vi "Alicat Full Driver Example.vi"() -> ()   [LabVIEW 2020]
doc: "Example program displaying the potential usage of nearly all of the VI's included in the Alicat LabVIEW Driver Library.\n\nThis VI only connects to a single Alicat at a time, and some features may be locked out due to circuit board revision or firmware revision (newer units have additional features available to them).\n\nIf you have any questions regarding the VI's used in this example, please see the Alicat LabVIEW Driver Library Manual (available on the Alicat website and included in the driver library. If you have remaining questions, please contact Alicat at (520) 290-6060 or info@alicat.com."
panel:
  in  "Tare AP Sensor":bool
  in  "Wait message":cluster{"Boolean":bool}
  in  "Read/Write Options":T1 {"Controller Select" items=["No controller"=0, "Volumetric Flow"=36, "Mass Flow"=37, "Absolute Pressure"=34, "Gauge Pressure"=38, "Differential Pressure"=39]}
  out "Batch Units":string="SL"
  in  "Serial Only":T2={"Valve Drive"=FALSE, "Totalizer"=TRUE, "Totalizer Timer"=FALSE, "Totalizer Peak Flow"=FALSE, "Show Abs., Gauge\nand Baro. pressures"=FALSE}
  in  "Data Logging Options":T3={"Absolute Press."=TRUE, "Gauge/Diff. Press."=TRUE, "Barometric Press."=TRUE, "Temperature"=TRUE, "Volumetric"=TRUE, "Mass Flow"=TRUE, "Setpoint"=TRUE, "Valve Drive"=FALSE, "Totalizer"=TRUE, "Tot. Timer [s]"=FALSE, "Tot. Avg. Flow"=FALSE, "Tot. Peak Flow"=FALSE, "Gas Selected"=TRUE, "Log Data"=FALSE}
  out "Measurement Data":T4
  in  "Chart: Manual Scale Adjust":bool
  in  "Chart: AutoScale":bool=TRUE
  out "Chart":T5(graph)
  out "Register value":string
  in  "Reg. to read":u16
  in  "Read Register":bool
  in  "COMPOSER gas mix input":T6={"Mix % 1"=0.0, "Include # 1"=FALSE, "Mix % 2"=0.0, "Include # 2"=FALSE, "Mix % 3"=0.0, "Include # 3"=FALSE, "Mix % 4"=0.0, "Include # 4"=FALSE, "Mix % 5"=0.0, "Include # 5"=FALSE, "COMPOSER gas 1"=0, "COMPOSER gas 2"=0, "COMPOSER gas 3"=0, "COMPOSER gas 4"=0, "COMPOSER gas 5"=0, "Create COMPOSER Mix"=FALSE, "Mix #"=236, "Mix name"="MyMix1", "Completion\ntext"="", "Create COMPOSER Mix 2"=FALSE} {"Mix #" min=236 max=255 step=1; "Mix % 1" min=0.0 max=100.0 step=0.01; "Mix % 2" min=0.0 max=100.0 step=0.01; "Mix % 3" min=0.0 max=100.0 step=0.01; "Mix % 4" min=0.0 max=100.0 step=0.01; "Mix % 5" min=0.0 max=100.0 step=0.01}
  in  "Chart: Setpoint":bool=TRUE
  in  "PID Settings":T7 {"P Gain" min=0 max=65535 step=1; "D Gain" min=0 max=65535 step=1; "I Gain" min=0 max=65535 step=1}
  in  "Log Register Values":bool
  out "Meas. per\nsecond [Hz]":dbl caption="Elapsed Time (s)"
  out "Time between\nreadings [ms]":dbl caption="Elapsed Time (s)"
  in  "Chart: Graphing":bool=TRUE
  out "Read-Only Options":T8={"Analog SP"=enum."4-20mA", "Control Invert"=enum."Pressure", "Main PWM"=enum."Volumetric Flow 0-2.5-5V bidir", "Aux PWM"=enum."Fixed 0.00V"}
  in  "Tare Options":T9={"Display"=enum."None", "External"=enum."None", "Auto-Tare Delay [s]"=nan} {"Auto-Tare Delay [s]" min=0.0 max=25.5 step=0.1 format="%.1g"}
  in  "Tare Pressure":bool
  in  "Tare Flow":bool
  in  "Reset Total":bool
  in  "Chart: Mass Flow":bool=TRUE
  in  "Chart: Volumetric":bool=TRUE
  in  "Chart: Temperature":bool=TRUE
  in  "Chart: Pressure":bool=TRUE
  in  "Time between \nreadings [ms]":u32
  out "Totalizer":T10(ring)
  out "Setpoint Units":string="SLPM"
  in  "Serial and Display":T11={"Pressure"=TRUE, "Temperature"=TRUE, "Volumetric"=TRUE, "Mass Flow"=TRUE, "Tot. Avg Flow"=FALSE, "Gas Selected"=TRUE}
  out "(Full Scale)":dbl=nan
  in  "Setpoint":dbl
  in  "Batch Setpoint":dbl format="%.3f"
  in  "Gas Select":u16(ring)
  out "Manufacturer Info":string
  in  "COM Port Settings":T12={"Unit ID"="A", "Baud Rate"=enum."19200", "VISA Sesssion In"="COM1"}
  # "Setpoint and Batching Controls"
  # "Manual Tare"
  # "Data Frame Enables"
  # "Controller Options\nand Analog Signal\nInformation"
  # "(Resetting the Totalizer will reset the batch)"
  # "Graphing Options:"
  # "VI Timing Options"
  # "Register Values"
  # "Populating VI with device information, please wait."
  # "Altering log options will start a new data log"
  # "(The data will be logged to the folder containing the VI)"
  # "Totalizer Timer"
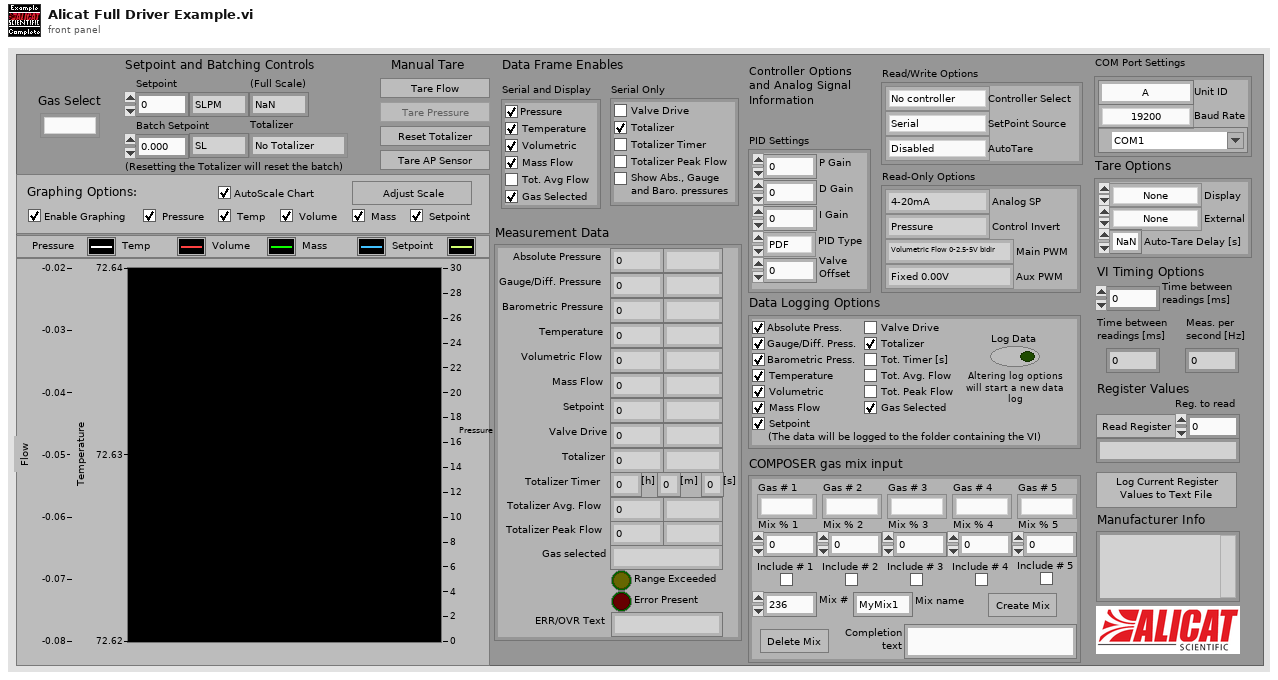
[diagram p1: front panel]
types:
  T1 = cluster{"Controller Select":u16, "SetPoint Source":enum8{"Serial", "Local", "Analog", "Unknown"}, "AutoTare":enum16{"Disabled", "Enabled"}}
  T2 = cluster{"Valve Drive":bool, "Totalizer":bool, "Totalizer Timer":bool, "Totalizer Peak Flow":bool, "Show Abs., Gauge\nand Baro. pressures":bool}
  T3 = cluster{"Absolute Press.":bool, "Gauge/Diff. Press.":bool, "Barometric Press.":bool, "Temperature":bool, "Volumetric":bool, "Mass Flow":bool, "Setpoint":bool, "Valve Drive":bool, "Totalizer":bool, "Tot. Timer [s]":bool, "Tot. Avg. Flow":bool, "Tot. Peak Flow":bool, "Gas Selected":bool, "Log Data":bool}
  T4 = cluster{"Absolute Pressure":dbl, "Gauge/Diff. Pressure":dbl, "Barometric Pressure":dbl, "Temperature":dbl, "Volumetric Flow":dbl, "Mass Flow":dbl, "Setpoint":dbl, "Valve Drive":dbl, "Totalizer":dbl, "[h]":dbl, "[m]":dbl, "[s]":dbl, "Totalizer Avg. Flow":dbl, "Totalizer Peak Flow":dbl, "Gas selected":string, "Range Exceeded":bool, "Error Present":bool, "ERR/OVR Text":string, "Abs. Pressure":string, "Temperature 2":string, "Volume":string, "Mass":string, "Totalizer 2":string, "Valve Drive 2":string, "Gauge/Diff. Press.":string, "Barometric Press.":string, "Setpoint 2":string, "Tot. Avg. Flow":string, "Tot. Peak Flow":string}
  T5 = cluster{"Pressure":dbl, "Temperature":dbl, "Volumetric":dbl, "Mass":dbl, "SetPoint":dbl}
  T6 = cluster{"Mix % 1":dbl, "Include # 1":bool, "Mix % 2":dbl, "Include # 2":bool, "Mix % 3":dbl, "Include # 3":bool, "Mix % 4":dbl, "Include # 4":bool, "Mix % 5":dbl, "Include # 5":bool, "COMPOSER gas 1":u16, "COMPOSER gas 2":u16, "COMPOSER gas 3":u16, "COMPOSER gas 4":u16, "COMPOSER gas 5":u16, "Create COMPOSER Mix":bool, "Mix #":u16, "Mix name":string, "Completion\ntext":string, "Create COMPOSER Mix 2":bool}
  T7 = cluster{"P Gain":i32, "D Gain":i32, "I Gain":i32, "PID Type":enum8{"PDF", "PD2I"}, "Valve \nOffset":i32}
  T8 = cluster{"Analog SP":enum16{"0-5V", "4-20mA"}, "Control Invert":enum16{"Pressure", "Vacuum/BP"}, "Main PWM":enum8{"Fixed 0.00V", "Pressure 0-5V", "Temperature 0-5V", "Volumetric Flow 0-5V", "Mass Flow 0-5V", "Pressure 0-2.5-5V bidir", "Temperature 0-2.5-5V bidir", "Volumetric Flow 0-2.5-5V bidir", "Mass Flow 0-2.5-5V bidir", "Pressure 1-5V", "Temperature 1-5V", "Volumetric Flow 1-5V", "Mass Flow 1-5V", "Reserved(A)", "Reserved(B)", "Fixed 5.12V"}, "Aux PWM":enum8{"Fixed 0.00V", "Pressure 0-5V", "Temperature 0-5V", "Volumetric Flow 0-5V", "Mass Flow 0-5V", "Pressure 0-2.5-5V bidir", "Temperature 0-2.5-5V bidir", "Volumetric Flow 0-2.5-5V bidir", "Mass Flow 0-2.5-5V bidir", "Pressure 1-5V", "Temperature 1-5V", "Volumetric Flow 1-5V", "Mass Flow 1-5V", "Reserved(A)", "Reserved(B)", "Fixed 5.12V"}}
  T9 = cluster{"Display":enum16{"None", "Pressure", "Volumetric"}, "External":enum16{"None", "Pressure", "Volumetric", "Totalizer"}, "Auto-Tare Delay [s]":dbl}
  T10 = enum8{"No Totalizer", "Mass Flow", "Volumetric Flow"}
  T11 = cluster{"Pressure":bool, "Temperature":bool, "Volumetric":bool, "Mass Flow":bool, "Tot. Avg Flow":bool, "Gas Selected":bool}
  T12 = cluster{"Unit ID":string, "Baud Rate":enum8{"2400", "9600", "19200", "38400", "57600", "115200", "Unknown"}, "VISA Sesssion In":refnum<visa-resource-name>}
  T13 = cluster{"Absolute Pressure":bool, "Gauge/Diff. Pressure":bool, "Barometric Pressure":bool, "Temperature":bool, "Volumetric":bool, "Mass":bool, "Setpoint":bool, "Valve Drive":bool, "Totalizer":bool, "Totalizer Timer":bool, "Totalizer Average Flow":bool, "Totalizer Peak Flow":bool, "Gas Selected":bool, "Tot. Timer Format":u16}
  T14 = cluster{"Controller Full Scale":dbl, "Controller Select":u16, "Control Range":enum16{"Normal", "Inverted", "Bidirectional", "Unknown"}}
  T15 = cluster{"Absolute Pressure":dbl, "Gauge/Diff. Pressure":dbl, "Barometric Pressure":dbl, "Temperature":dbl, "Volumetric Flow":dbl, "Mass Flow":dbl, "Setpoint":dbl, "Valve Drive":dbl, "Totalizer":dbl, "[h]":dbl, "[m]":dbl, "[s]":dbl, "Totalizer Average Flow":dbl, "Totalizer Peak Flow":dbl, "Gas selected":string, "Range Exceeded":bool, "Error Present":bool, "ERR/OVR Text":string, "Abs. Pressure":string, "Temperature 2":string, "Volume":string, "Mass":string, "Totalizer 2":string, "Valve Drive 2":string, "Gauge/Diff. Press.":string, "Barometric Press.":string, "Setpoint 2":string, "Tot. Avg. Flow":string, "Tot. Peak Flow":string}
  T16 = cluster{"Abs. Pressure":string, "Gauge/Diff. Press.":string, "Barometric Press.":string, "Temperature":string, "Volume":string, "Mass":string, "Setpoint":string, "Valve Drive":string, "Totalizer":string, "Tot. Timer":string, "Tot. Avg. Flow":string, "Tot. Peak Flow":string}
  T17 = cluster{"Pressure":bool, "Temperature":bool, "Volumetric":bool, "Mass Flow":bool, "Setpoint":bool, "Chart: AutoScale":bool}
  T18 = cluster{"Enabled":enum8{"Enabled", "Disabled", "Disabled and Grayed Out"}, "Disabled and Grayed Out":enum8{"Enabled", "Disabled", "Disabled and Grayed Out"}}
  T19 = cluster{"Absolute Pressure":dbl, "Gauge/Diff. Pressure":dbl, "Barometric Pressure":dbl, "Temperature":dbl, "Volumetric":dbl, "Mass Flow":dbl, "Setpoint":dbl, "Valve Drive":dbl, "Totalizer":dbl, "[hr]":dbl, "[min]":dbl, "[sec]":dbl, "Totalizer Average Flow":dbl, "Totalizer Peak Flow":dbl, "Gas selected":string}
  T20 = cluster{"Pressure(s)":bool, "Temperature":bool, "Volumetric":bool, "Mass":bool, "Totalizer Average Flow":bool, "Gas Selected":bool}
  T21 = enum16{"open", "replace", "create", "open or create", "replace or create", "replace or create with confirmation"}
  T22 = cluster{"P Gain":i32, "D Gain":i32, "I Gain":i32}
  T23 = cluster{"PID Type":enum8{"PDF", "PD2I"}, "Valve Offset":i32}
  T24 = cluster{"Gas # 1":u16, "Mix % 1":dbl, "Include # 1":bool, "Gas # 2":u16, "Mix % 2":dbl, "Include # 2":bool, "Gas # 3":u16, "Mix % 3":dbl, "Include # 3":bool, "Gas # 4":u16, "Mix % 4":dbl, "Include # 4":bool, "Gas # 5":u16, "Mix % 5":dbl, "Include # 5":bool}
  T25 = cluster{"Pressure":bool, "Temperature":bool, "Volumetric":bool, "Mass":bool, "Totalizer Average Flow":bool, "Gas Selected":bool}
  T26 = enum8{"Enabled", "Disabled", "Disabled and Grayed Out"}
  T27 = typedef "Data Frame.ctl" = cluster{"Absolute Pressure":bool, "Gauge/Diff. Pressure":bool, "Barometric Pressure":bool, "Temperature":bool, "Volumetric":bool, "Mass":bool, "Setpoint":bool, "Valve Drive":bool, "Totalizer":bool, "Totalizer Timer":bool, "Totalizer Average Flow":bool, "Totalizer Peak Flow":bool, "Gas Selected":bool, "Tot. Timer Format":u16}
  T28 = enum16{"None", "Pressure", "Volumetric", "Totalizer"}
  T29 = cluster{"Valve Amount":enum8{"Single Valve", "Dual Valve"}, "PID Type":enum8{"PDF", "PD2I"}, "Valve Offset":i32, "P Gain":i32, "D Gain":i32, "I Gain":i32}
  T30 = cluster{"Absolute Pressure":dbl, "Gauge/Diff. Pressure":dbl, "Volumetric Flow":dbl, "Mass Flow":dbl}
  T31 = typedef "Data Cluster.ctl" = cluster{"Absolute Pressure":dbl, "Gauge/Diff. Pressure":dbl, "Barometric Pressure":dbl, "Temperature":dbl, "Volumetric Flow":dbl, "Mass Flow":dbl, "Setpoint":dbl, "Valve Drive":dbl, "Totalizer":dbl, "[hr]":dbl, "[min]":dbl, "[sec]":dbl, "Totalizer Average Flow":dbl, "Totalizer Peak Flow":dbl, "Gas selected":string}
  T32 = enum8{"2400", "9600", "19200", "38400", "57600", "115200", "Unknown"}
  T33 = cluster{"Absolute Pressure":dbl, "Gauge/Diff. Pressure":dbl, "Barometric Pressure":dbl, "Temperature":dbl, "Volumetric Flow":dbl, "Mass Flow":dbl, "Setpoint":dbl, "Valve Drive":dbl, "Totalizer":dbl, "[hr]":dbl, "[min]":dbl, "[sec]":dbl, "Totalizer Average Flow":dbl, "Totalizer Peak Flow":dbl, "Gas selected":string}
  T34 = cluster{"Pressure":bool, "Temperature":bool, "Volumetric":bool, bool, bool, "Gas Selected":bool}
  T35 = enum16{"Left Button", "Center Button", "Right Button", "Window Close"}
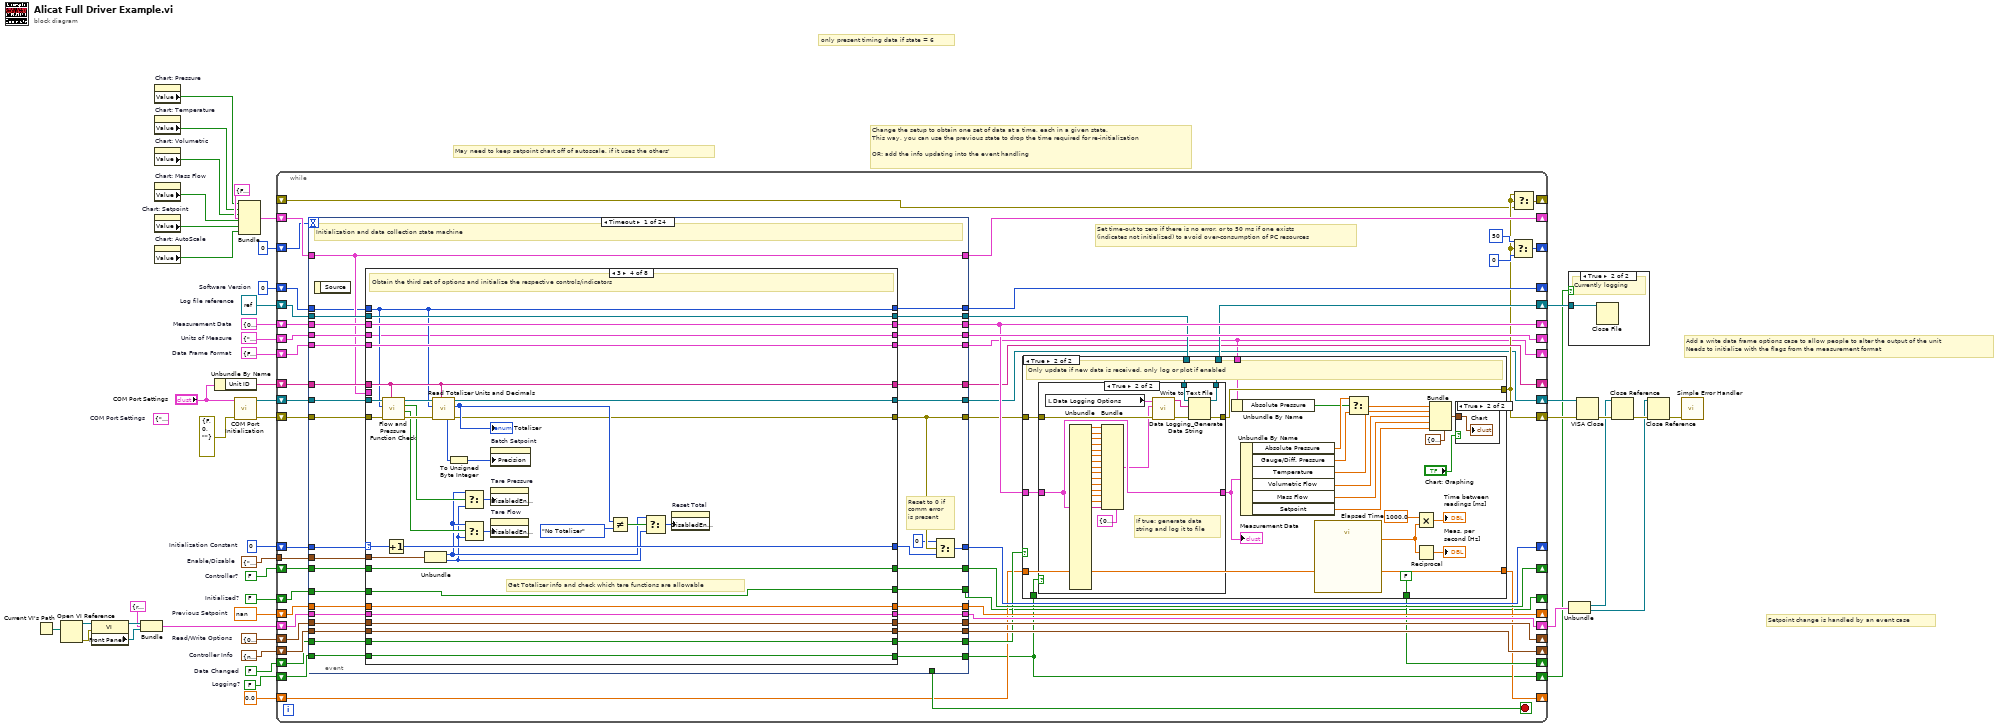
[diagram p0: block diagram]
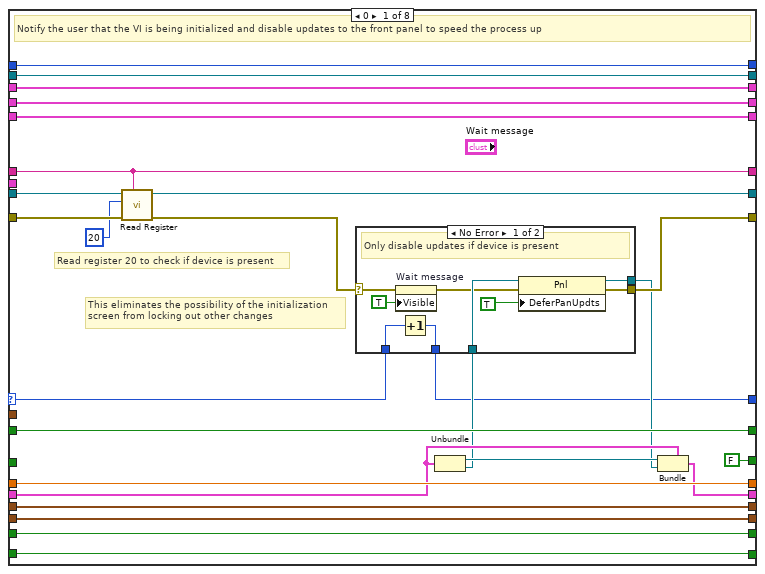
[diagram p6: hidden frame]
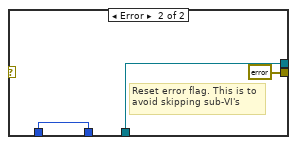
[diagram p7: hidden frame]
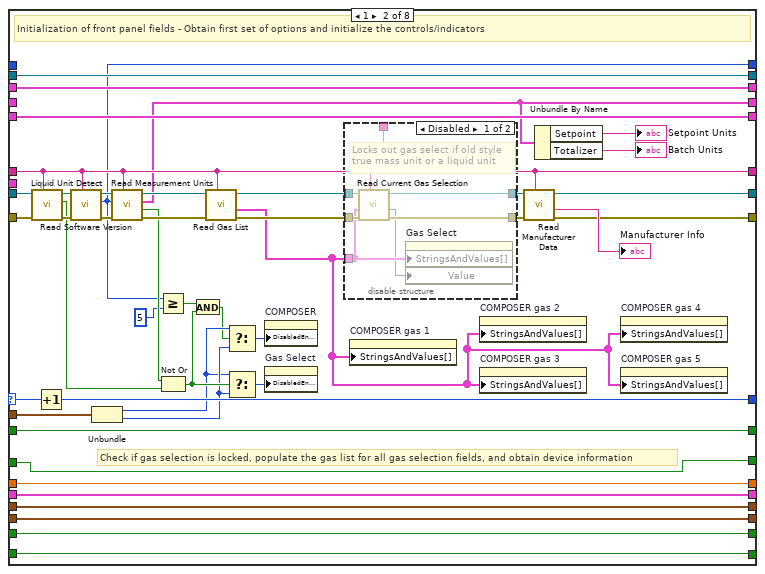
[diagram p8: hidden frame]
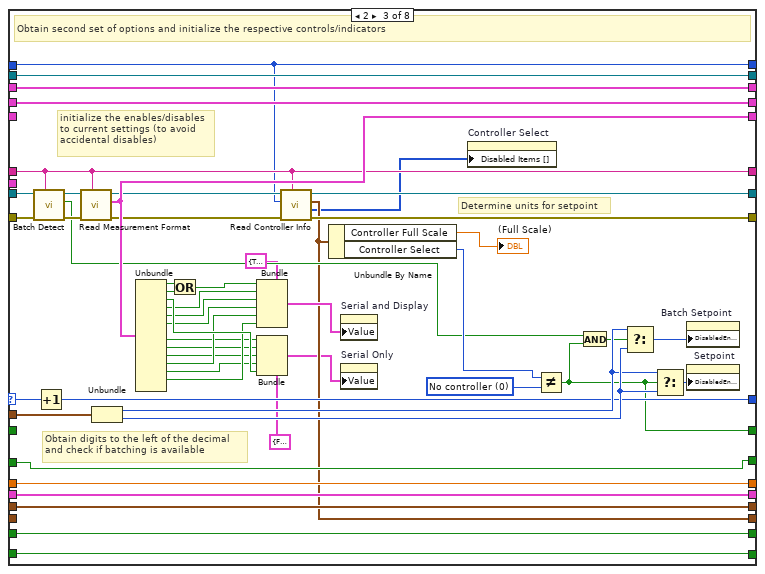
[diagram p10: hidden frame]
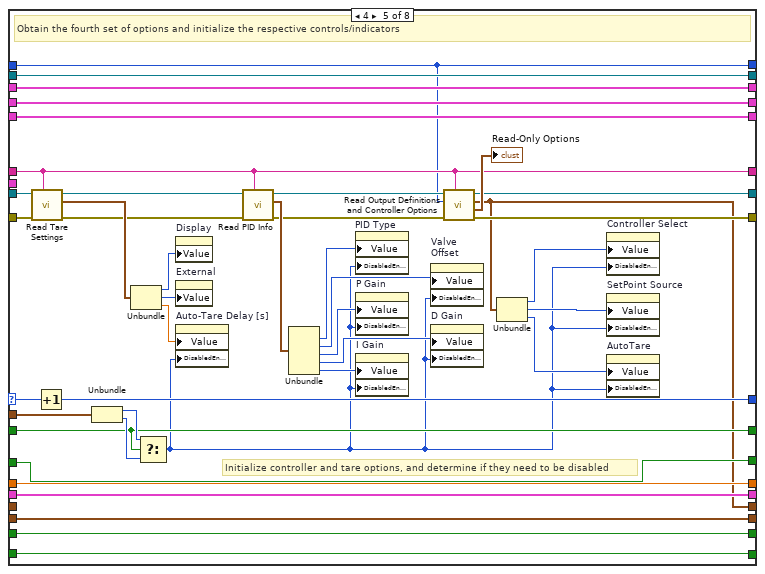
[diagram p11: hidden frame]
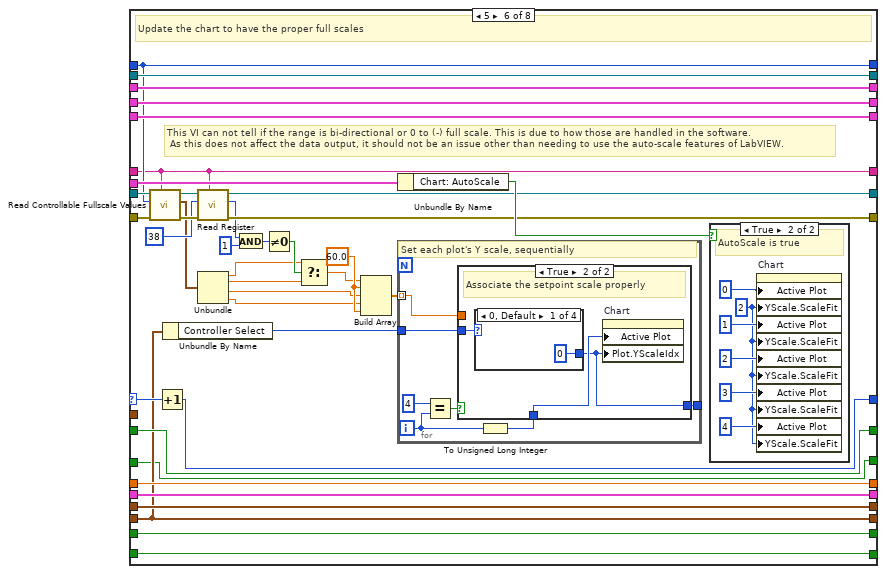
[diagram p12: hidden frame]
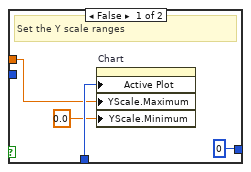
[diagram p14: hidden frame]
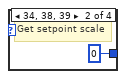
[diagram p15: hidden frame]
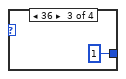
[diagram p16: hidden frame]
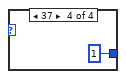
[diagram p17: hidden frame]
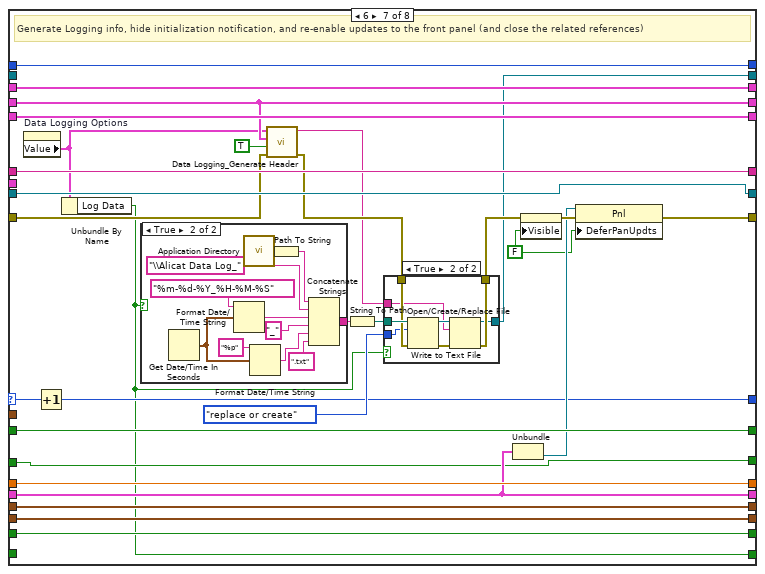
[diagram p18: hidden frame]
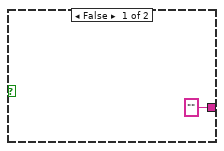
[diagram p19: hidden frame]
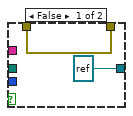
[diagram p20: hidden frame]
diagram:
  w1 = T13 {"Absolute Pressure"=FALSE, "Gauge/Diff. Pressure"=FALSE, "Barometric Pressure"=FALSE, "Temperature"=FALSE, "Volumetric"=FALSE, "Mass"=FALSE, "Setpoint"=FALSE, "Valve Drive"=FALSE, "Totalizer"=FALSE, "Totalizer Timer"=FALSE, "Totalizer Average Flow"=FALSE, "Totalizer Peak Flow"=FALSE, "Gas Selected"=FALSE, "Tot. Timer Format"=0}  # Data Frame Format
  w2 = T1 {"Controller Select"=0, "SetPoint Source"=enum."Serial", "AutoTare"=enum."Disabled"}  # Read/Write Options
  w3 = T14 {"Controller Full Scale"=nan, "Controller Select"=0, "Control Range"=enum."Normal"}  # Controller Info
  (unwired) T12 {"Unit ID"="A", "Baud Rate"=enum."19200", "VISA Sesssion In"="COM1"}  # COM Port Settings
  w4 = T15 {"Absolute Pressure"=0.0, "Gauge/Diff. Pressure"=0.0, "Barometric Pressure"=0.0, "Temperature"=0.0, "Volumetric Flow"=0.0, "Mass Flow"=0.0, "Setpoint"=0.0, "Valve Drive"=0.0, "Totalizer"=0.0, "[h]"=0.0, "[m]"=0.0, "[s]"=0.0, "Totalizer Average Flow"=0.0, "Totalizer Peak Flow"=0.0, "Gas selected"="", "Range Exceeded"=FALSE, "Error Present"=FALSE, "ERR/OVR Text"="", "Abs. Pressure"="", "Temperature 2"="", "Volume"="", "Mass"="", "Totalizer 2"="", "Valve Drive 2"="", "Gauge/Diff. Press."="", "Barometric Press."="", "Setpoint 2"="", "Tot. Avg. Flow"="", "Tot. Peak Flow"=""}  # Measurement Data
  w5 = T16 {"Abs. Pressure"="", "Gauge/Diff. Press."="", "Barometric Press."="", "Temperature"="", "Volume"="", "Mass"="", "Setpoint"="", "Valve Drive"="", "Totalizer"="", "Tot. Timer"="", "Tot. Avg. Flow"="", "Tot. Peak Flow"=""}  # Units of Measure
  w6 = u8 0  # Software Version
  w8 = FALSE  # Logging?
  w9 = FALSE  # Initialized?
  w25 = FALSE  # Data Changed
  w27 = refnum<file> refnum  # Log file reference
  w37 = nan  # Previous Setpoint
  w38 = FALSE  # Controller?
  w39 = T18 {"Enabled"=enum."Enabled", "Disabled and Grayed Out"=enum."Disabled and Grayed Out"}  # Enable/Disable
  w40 = 0  # Initialization Constant
  # "May need to keep setpoint chart off of autoscale, if it uses the others'"
  # "only present timing data if state = 6"
  # "Change the setup to obtain one set of data at a time, each in a given state.\nThis way, you can use the previous state to drop the time required for re-initialization\n\nOR: add the info updating into the event handling"
  # "Setpoint change is handled by an event case"
  # "Add a write data frame options case to allow people to alter the output of the unit\nNeeds to initialize with the flags from the measurement format"
  n1 = Current VI's Path() -> (path=w34:path)
  n2 = Open VI Reference(vi path=w34) -> (vi reference=w32:refnum<vi>, error out=w33:errorcluster)  [unwired: 2 in, 3 out]
  n3 = property class="VI"(reference=w32, error in=w33) -> (reference out=w30:refnum<vi>, "Front Panel"=w31:refnum<vi>)  [unwired: 1 out]
  n4 = Bundle(cluster=cluster{refnum<vi>, "Panel":refnum<vi>} {refnum, "Panel"=refnum}, w30, "Panel"=w31) -> (w29:cluster{refnum<vi>, "Panel":refnum<vi>})
  n5 = property on="Chart: Pressure" class="Bool (strict)"() -> ("Value"=w19:bool)  [unwired: 2 in, 2 out]
  n6 = property on="Chart: Temperature" class="Bool (strict)"() -> ("Value"=w20:bool)  [unwired: 2 in, 2 out]
  n7 = property on="Chart: Volumetric" class="Bool (strict)"() -> ("Value"=w21:bool)  [unwired: 2 in, 2 out]
  n8 = property on="Chart: Mass Flow" class="Bool (strict)"() -> ("Value"=w22:bool)  [unwired: 2 in, 2 out]
  n9 = property on="Chart: Setpoint" class="Bool (strict)"() -> ("Value"=w23:bool)  [unwired: 2 in, 2 out]
  n10 = property on="Chart: AutoScale" class="Bool (strict)"() -> ("Value"=w17:bool)  [unwired: 2 in, 2 out]
  n11 = Unbundle By Name("COM Port Settings") -> ("Unit ID"=w41:string)
  n12 = call "COM Port Initialization.vi"("error in (no error)"=errorcluster {"status"=FALSE, "code"=0, "source"=""}, "Communication Settings"="COM Port Settings") -> ("error out"=w44:errorcluster, "VISA Session Out"=w46:refnum<visa-resource-name>)  [unwired: 8 in]
  n13 = Bundle(cluster=T17 {"Pressure"=FALSE, "Temperature"=FALSE, "Volumetric"=FALSE, "Mass Flow"=FALSE, "Setpoint"=FALSE, "Chart: AutoScale"=TRUE} ("Graphing enables"), "Pressure"=w19, "Temperature"=w20, "Volumetric"=w21, "Mass Flow"=w22, "Setpoint"=w23, "Chart: AutoScale"=w17) -> (w35:T17)
  n14 = while {
    shift-right: [w91] -> _
    shift-left: w40 -> [w92]
    shift-right: [w73] -> _
    shift-left: w4 -> [w90]
    shift-right: [w88] -> _
    shift-left: w5 -> [w89]
    tunnel: w39 -> [w87]
    shift-right: [w47] -> _
    shift-left: w1 -> [w86]
    shift-right: [w48] -> w45
    shift-left: w46 -> [w95]
    shift-right: [w51] -> w43
    shift-left: w44 -> [w94]
    shift-right: [w52] -> _
    shift-left: w41 -> [w93]
    shift-right: [w85] -> _
    shift-left: w38 -> [w84]
    shift-right: [w83] -> _
    shift-left: w37 -> [w82]
    shift-right: [w63] -> _
    shift-left: w35 -> [w64]
    shift-right: [w80] -> w12
    shift-left: w29 -> [w81]
    shift-right: [w77] -> _
    shift-left: w2 -> [w78]
    shift-right: [w75] -> _
    shift-left: w3 -> [w76]
    shift-right: [w67] -> w26
    shift-left: w27 -> [w74]
    shift-right: [w71] -> _
    shift-left: w25 -> [w72]
    shift-right: [w66] -> _
    shift-left: 0.0 ("Get Start Time (s)") -> [w65]
    shift-right: [w59] -> _
    shift-left: 0 -> [w60]
    shift-right: [w57] -> _
    shift-left: w9 -> [w58]
    shift-right: [w55] -> w7
    shift-left: w8 -> [w56]
    shift-right: [w54] -> _
    shift-left: w6 -> [w53]
    shift-right: [w50] -> _
    shift-left: _ -> [w49]
    stop <- w79 stop-if-true
    # "Set time-out to zero if there is no error, or to 50 ms if one exists\n(indicates not initialized) to avoid over-consumption of PC resources"
    n15 = event shown="[0] Timeout" {
      selector: _ -> [_ _ _ _ _ _ _ _ _ _ _ _ _ _ _ _ _ _ _ _ _ _ _ _]
      dyn-events: _ -> [_ _ _ _ _ _ _ _ _ _ _ _ _ _ _ _ _ _ _ _ _ _ _ _]
      timeout: w60 -> [_ _ _ _ _ _ _ _ _ _ _ _ _ _ _ _ _ _ _ _ _ _ _ _]
      tunnel: [w188 w594 w616 w634 w663 w679 w700 w721 w742 w765 w787 w821 w845 w878 w893 w951 w980 w1006 w1024 w1116 w1146 w1166 w1215 w1268] -> w48
      tunnel: w95 -> [w192 w594 w612 w635 w663 w678 w699 w720 w741 w766 w788 w810 w851 w871 w923 w952 w981 w996 w1073 w1120 w1146 w1166 w1215 w1268]
      tunnel: w94 -> [w191 w593 w613 w637 w662 w681 w702 w723 w744 w763 w785 w830 w852 w870 w922 w949 w979 w995 w1072 w1119 w1147 w1167 w1205 w1251]
      tunnel: [w171 w593 w617 w636 w662 w680 w701 w722 w743 w764 w786 w820 w844 w877 w888 w950 w967 w1004 w1063 w1096 w1147 w1167 w1196 w1265] -> w69
      tunnel: w93 -> [w190 w595 w622 w643 _ w677 w698 w719 w740 w761 w784 w805 w843 w876 w892 w948 w978 w991 w1023 w1113 w1145 w1165 w1214 w1267]
      tunnel: w92 -> [w189 w592 _ _ _ w682 w703 w724 w745 w767 w789 w822 w853 w879 w924 w953 w982 w1007 w1074 w1121 w1150 w1170 w1218 w1271]
      tunnel: [w172 w592 0 ("Initialization Constant") 0 ("Initialization Constant") 0 ("t") w683 w704 w725 w746 w768 w790 w823 w854 w880 w925 w954 w983 w1008 w1075 w1122 w1151 w1171 w1219 w1272] -> w91
      tunnel: w90 -> [w187 w598 w624 w645 w669 w690 w711 w732 w753 w775 w797 w829 w861 w887 w932 w961 w990 w1015 w1022 w1128 w1157 w1177 w1225 w1277]
      tunnel: [w178 w598 w624 w645 w669 w690 w711 w732 w753 w775 w797 w829 w861 w887 w932 w961 w990 w1015 w1021 w1128 w1157 w1177 w1225 w1277] -> w73
      tunnel: w89 -> [w186 w597 w623 w644 w668 w689 w710 w731 w752 w774 w796 w828 w860 w886 w931 w960 w989 w1014 w1030 w1127 w1156 w1176 w1224 w1259]
      tunnel: [w185 w597 w623 w644 w668 w689 w710 w731 w752 w774 w796 w828 w860 w886 w931 w960 w989 w1014 w1030 w1127 w1156 w1176 w1224 w1259] -> w88
      tunnel: w87 -> [w184 _ _ _ _ _ _ _ _ _ _ _ _ _ _ _ _ _ _ _ _ _ _ _]
      tunnel: w86 -> [w183 w596 w621 w642 w667 w688 w709 w730 w751 w773 w795 w827 w859 w885 w930 w959 w988 w1013 w1019 _ w1144 w1164 w1191 w1256]
      tunnel: [w182 w595 w622 w643 w660 w677 w698 w719 w740 w761 w784 w805 w843 w876 w892 w948 w978 w991 w1023 w1113 w1145 w1165 w1214 w1267] -> w52
      tunnel: [w181 w596 w621 w642 w667 w688 w709 w730 w751 w773 w795 w827 w859 w885 w930 w959 w988 w1013 w1018 w1111 w1144 w1164 w1191 w1256] -> w47
      tunnel: [w180 w591 w620 w641 w666 w687 w708 w729 w750 w772 w794 w806 w858 w884 w929 w958 w987 w1012 w1078 w1126 w1155 w1175 w1223 w1276] -> w85
      tunnel: w84 -> [w179 w591 w620 w641 w666 w687 w708 w729 w750 w772 w794 w806 w858 w884 w929 w958 w987 w1012 w1078 w1126 w1155 w1175 w1223 w1276]
      tunnel: w82 -> [w177 w590 w619 w640 w665 w686 w707 w728 w749 w771 w793 w826 w857 w883 w928 w957 w986 w1011 w1070 w1125 w1154 w1174 w1222 w1275]
      tunnel: [w176 w590 w619 w640 w665 w686 w707 w728 w749 w771 w793 w826 w857 w883 w928 w957 w986 w1011 w1017 w1125 w1154 w1174 w1222 w1275] -> w83
      tunnel: w81 -> [w175 w589 w618 w639 w664 w685 w706 w727 w748 w770 w792 w825 w856 w882 w927 w956 w985 w1010 w1077 w1124 w1153 w1173 w1221 w1274]
      tunnel: [w174 w589 w618 w639 w664 w685 w706 w727 w748 w770 w792 w825 w856 w882 w927 w956 w985 w1010 w1077 w1124 w1153 w1173 w1221 w1274] -> w80
      tunnel: [_ w599 _ _ _ _ _ _ _ _ _ _ _ _ _ _ _ _ _ _ _ _ _ _] -> w79
      tunnel: w78 -> [w169 w588 w611 w631 w659 w676 w697 w718 w739 w760 w782 w819 w842 w868 w900 w939 w977 w1005 w1071 w1118 w1149 w1169 w1217 w1270]
      tunnel: [w168 w588 w611 w631 w659 w676 w697 w718 w739 w760 w782 w816 w842 w868 w900 w939 w977 w1005 w1071 w1118 w1149 w1169 w1217 w1270] -> w77
      tunnel: w76 -> [w167 w587 w610 w630 w658 w675 w696 w717 w738 w759 w781 w815 w841 w867 w899 w938 w976 w1002 w1065 w1117 w1148 w1168 w1216 w1269]
      tunnel: [w166 w587 w610 w630 w658 w675 w696 w717 w738 w759 w781 w815 w841 w867 w899 w938 w976 w1002 w1064 w1117 w1148 w1168 w1216 w1269] -> w75
      tunnel: [w165 w586 w609 w629 w657 w674 w695 w716 w737 w758 w780 w814 w840 w866 w898 w937 w966 w1001 w1062 w1110 w1143 w1163 w1213 w1260] -> w68
      tunnel: w74 -> [w164 w586 w609 w629 w657 w674 w695 w716 w737 w758 w780 w814 w840 w866 w898 w937 w966 w1001 w1062 w1110 w1143 w1163 w1213 w1252]
      tunnel: w72 -> [w163 _ _ _ _ _ _ _ _ _ _ _ _ _ _ _ _ _ _ _ _ _ _ _]
      tunnel: [w162 _ _ _ _ _ _ _ _ _ _ _ _ _ _ _ _ _ TRUE ("Data Changed") _ _ _ _ _] -> w70
      tunnel: w64 -> [w161 w585 w608 w628 w656 w673 w694 w715 w736 w757 w779 w804 w839 w865 w897 w936 w965 w1000 w1059 w1108 w1142 w1162 w1212 w1255]
      tunnel: [w161 w585 w608 w628 w656 w673 w694 w715 w736 w757 w779 w804 w839 w865 w897 w936 w965 w1000 w1059 w1108 w1142 w1162 w1212 w1255] -> w63
      tunnel: w58 -> [w160 w584 w607 w627 w655 w672 w693 w714 w735 w756 w778 w803 w838 w864 w896 w935 w964 w999 w1058 w1107 w1131 w1160 w1193 w1254]
      tunnel: [w159 w584 w607 w627 w655 w672 w693 w714 w735 w756 w778 w803 w838 w864 w896 w935 w964 w999 w1058 w1107 w1131 w1160 w1193 w1254] -> w57
      tunnel: w56 -> [w158 w583 w606 w626 w654 w671 w692 w713 w734 w755 w777 w802 w837 w863 w891 w934 w963 w998 w1057 w1098 w1130 w1159 w1192 w1249]
      tunnel: [w157 w583 w606 w626 w654 w671 w692 w713 w734 w755 w777 w802 w837 w863 w891 w934 w963 w998 w1057 w1098 w1130 w1159 w1192 w1253] -> w55
      tunnel: [w156 w582 w605 w625 w653 w670 w691 w712 w733 w754 w776 w800 w835 w862 w890 w933 w962 w997 w1016 w1095 w1129 w1158 w1190 w1247] -> w54
      tunnel: w53 -> [w155 w582 w605 w625 w653 w670 w691 w712 w733 w754 w776 w800 w835 w862 w890 w933 w962 w997 w1016 w1095 w1129 w1158 w1190 w1247]
      event Timeout {
        # "Reset to 0 if\ncomm error\nis present"
        # "Initialization and data collection state machine"
        n16 = event-data() -> ()  [unwired: 1 in, 1 out]
        n17 = case shown="3" w189 {
          selector: w189 -> [w196 w275 w336 w351 w411 w443 w481 w555]
          tunnel: w192 -> [w206 w264 w305 w370 w390 w432 w503 w566]
          tunnel: w191 -> [w207 w263 w304 w371 w391 w431 w494 w565]
          tunnel: w190 -> [w204 w250 w324 w349 w399 w424 w502 w560]
          tunnel: [w195 w274 w319 w350 w409 w442 w482 w555] -> w173
          tunnel: [w205 w262 w325 w353 w386 w429 w503 w559] -> w188
          tunnel: [w213 w261 w326 w354 w387 w428 w483 w558] -> w171
          tunnel: w187 -> [w216 w260 w331 w356 w408 w449 w500 w579]
          tunnel: [w216 w260 w331 w356 w408 w449 w500 w578] -> w178
          tunnel: [w217 w233 w308 w337 w407 w450 w493 w563] -> w185
          tunnel: w186 -> [w217 _ w308 w337 w407 w450 w493 w563]
          tunnel: w184 -> [_ w259 w330 w363 w410 _ _ _]
          tunnel: [w218 w258 w329 w355 w406 w451 w501 w545] -> w181
          tunnel: w183 -> [w218 w258 _ w355 w406 w451 w501 w564]
          tunnel: [w204 w250 w324 w349 w399 w424 w502 w560] -> w182
          tunnel: [w215 w257 w315 w352 w392 w447 w504 w557] -> w180
          tunnel: w179 -> [w215 w257 _ w352 w392 w447 w504 w557]
          tunnel: w177 -> [w214 w256 w318 w348 w412 w446 w505 _]
          tunnel: [w214 w256 w318 w348 w412 w446 w505 w544] -> w176
          tunnel: w175 -> [w211 w255 w317 w347 w383 w445 w499 w553]
          tunnel: [w208 w255 w317 w347 w383 w445 w499 w553] -> w174
          tunnel: w169 -> [w201 w240 w313 w344 _ w444 w496 w551]
          tunnel: [w201 w240 w313 w344 w377 w444 w496 w551] -> w168
          tunnel: w167 -> [w200 w239 _ w343 w382 w441 w495 w552]
          tunnel: [w200 w239 w306 w343 w382 w441 w495 w552] -> w166
          tunnel: [w199 w238 w312 w342 w381 w448 w486 w550] -> w165
          tunnel: w164 -> [w199 w238 w312 w342 w381 w448 _ w550]
          tunnel: w163 -> [w198 w237 w311 w341 w380 w439 w484 w548]
          tunnel: [w198 w237 w311 w341 w380 w439 w484 w549] -> w162
          tunnel: w161 -> [_ _ _ _ _ w436 _ _]
          tunnel: w160 -> [_ w236 w310 w340 w379 w434 w480 _]
          tunnel: [FALSE ("Data Changed") w236 w310 w340 w379 w434 w480 w549] -> w159
          tunnel: w158 -> [w194 w235 w309 w339 w378 w433 _ w547]
          tunnel: [w194 w235 w309 w339 w378 w433 w479 w547] -> w157
          tunnel: [w193 w234 w307 w338 w376 w430 w477 w546] -> w156
          tunnel: w155 -> [w193 _ w307 w338 w376 w430 w477 w546]
          frame 0 {
            # "This eliminates the possibility of the initialization\nscreen from locking out other changes"
            # "Read register 20 to check if device is present"
            # "Notify the user that the VI is being initialized and disable updates to the front panel to speed the process up"
            n18 = call "Read Register.vi"("Unit ID (A)"=w204, "error in"=w207, "Register address"=u16 20, "VISA Session In"=w206) -> ("error out"=w203:errorcluster, "VISA Session Out"=w205:refnum<visa-resource-name>)  [unwired: 5 in, 1 out]
            n19 = Unbundle(w211) -> (w212:refnum<vi>, "Panel"=w209:refnum<vi>)
            n20 = case shown="No Error" w203 {
              selector: w203 -> [w221 _]
              tunnel: [w226 errorcluster {"status"=FALSE, "code"=0, "source"=""} ("error out")] -> w213
              tunnel: [w225 w230] -> w210
              tunnel: w209 -> [w224 w230]
              tunnel: w196 -> [w220 w228]
              tunnel: [w219 w228] -> w195
              frame No Error {
                # "Only disable updates if device is present"
                n21 = property on="Wait message" class="Clust (strict)"(error in=w221, "Visible"=TRUE) -> (error out=w222:errorcluster)  [unwired: 1 in, 1 out]
                n22 = Increment(x=w220) -> (x+1=w219:i32)
                n23 = property class="Pnl"(reference=w224, error in=w222, "DeferPanUpdts"=TRUE ("Defer Panel Updates")) -> (reference out=w225:refnum<vi>, error out=w226:errorcluster)
              }
              frame Error {
                # "Reset error flag. This is to\navoid skipping sub-VI's"
              }
            }
            n24 = Bundle(cluster=w211, w212, "Panel"=w210) -> (w208:cluster{refnum<vi>, "Panel":refnum<vi>})
          }
          frame 1 {
            # "Check if gas selection is locked, populate the gas list for all gas selection fields, and obtain device information"
            # "Initialization of front panel fields - Obtain first set of options and initialize the controls/indicators"
            n25 = call "Liquid Unit Detect.vi"("Unit ID (A)"=w250, "error in"=w263, "VISA Session In"=w264) -> ("error out"=w268:errorcluster, "Liquid Device"=w266:bool, "VISA Session Out"=w269:refnum<visa-resource-name>)  [unwired: 6 in]
            n26 = Increment(x=w275) -> (x+1=w274:i32)
            n27 = call "Read Software Version.vi"("Unit ID (A)"=w250, "error in"=w268, "VISA Session In"=w269) -> ("error out"=w272:errorcluster, "Software Version"=w234:u8, "VISA Session Out"=w273:refnum<visa-resource-name>)  [unwired: 6 in]
            n28 = Unbundle(w259) -> ("Enabled"=w242:T26, "Disabled and Grayed Out"=w243:T26)
            n29 = call "Read Measurement Units.vi"("Unit ID (A)"=w250, "error in"=w272, "Software Rev"=w234, "VISA Session In"=w273) -> ("error out"=w271:errorcluster, "Lock Gas Select"=w267:bool, "Measurement Units"=w233:T16, "VISA Session Out"=w270:refnum<visa-resource-name>)  [unwired: 4 in]
            n30 = Greater Or Equal?(x=w234, y=u8 5) -> (x >= y?=w247:bool)
            n31 = Not Or(1:w266, 2:w267) -> (0:w246:bool)
            n32 = And(x=w247, y=w246) -> (x .and. y?=w241:bool)
            n33 = call "Read Gas List.vi"("Unit ID (A)"=w250, "error in"=w271, "VISA Session In"=w270) -> ("error out"=w254:errorcluster, "Gas Selection: Strings and Values"=w249:cluster{"Gas Name":string, "Gas number":u16}[], "VISA Session Out"=w251:refnum<visa-resource-name>)  [unwired: 5 in, 1 out]
            n34 = Select(t=w242, s=w241, f=w243) -> (s? t:f=w244:T26)
            n35 = Select(t=w242, s=w246, f=w243) -> (s? t:f=w245:T26)
            n36 = property on="COMPOSER" class="Clust"("DisabledEnum"=w244) -> ()  [unwired: 2 in, 2 out]
            n37 = property on="Gas Select" class="Ring (strict)"("DisabledEnum"=w245) -> ()  [unwired: 2 in, 2 out]
            n38 = disable-structure shown="Disabled" {
              disable-tunnel: w254 -> [w282 w283]
              disable-tunnel: [w281 w283] -> w253
              disable-tunnel: [w280 w284] -> w252
              disable-tunnel: w251 -> [w279 w284]
              disable-tunnel: w250 -> [w278 _]
              disable-tunnel: w249 -> [w277 _]
              frame Disabled {
                # "Locks out gas select if old style\ntrue mass unit or a liquid unit"
                n39 = call "Read Current Gas Selection.vi"("Unit ID (A)"=w278, "error in"=w282, "Gas Selection: Strings and Values"=w277, "VISA Session In"=w279) -> ("error out"=w281:errorcluster, "Current Gas Selection (number)"=w276:u16, "VISA Session Out"=w280:refnum<visa-resource-name>)  [unwired: 4 in, 1 out]
                n40 = property on="Gas Select" class="Ring (strict)"("StringsAndValues[]"=w277, "Value"=w276) -> ()  [unwired: 2 in, 2 out]
              }
              frame Enabled {
              }
            }
            n41 = property on="COMPOSER gas 1" class="Ring (strict)"("StringsAndValues[]"=w249) -> ()  [unwired: 2 in, 2 out]
            n42 = property on="COMPOSER gas 2" class="Ring (strict)"("StringsAndValues[]"=w249) -> ()  [unwired: 2 in, 2 out]
            n43 = property on="COMPOSER gas 3" class="Ring (strict)"("StringsAndValues[]"=w249) -> ()  [unwired: 2 in, 2 out]
            n44 = call "Read Manufacturer Data.vi"("Unit ID (A)"=w250, "error in"=w253, "VISA Session In"=w252) -> ("error out"=w261:errorcluster, "Manufacturer Info"=→"Manufacturer Info":string, "VISA Session Out"=w262:refnum<visa-resource-name>)  [unwired: 6 in]
            n45 = Unbundle By Name(w233) -> ("Setpoint"=→"Setpoint Units":string, "Totalizer"=→"Batch Units":string)
            n46 = property on="COMPOSER gas 4" class="Ring (strict)"("StringsAndValues[]"=w249) -> ()  [unwired: 2 in, 2 out]
            n47 = property on="COMPOSER gas 5" class="Ring (strict)"("StringsAndValues[]"=w249) -> ()  [unwired: 2 in, 2 out]
          }
          frame 2 {
            w287 = u16 0 items=["No controller"=0, "Volumetric Flow"=36, "Mass Flow"=37, "Absolute Pressure"=34, "Gauge Pressure"=38, "Differential Pressure"=39] ("Controller Select")
            # "Obtain digits to the left of the decimal\nand check if batching is available"
            # "Determine units for setpoint"
            # "initialize the enables/disables\nto current settings (to avoid \naccidental disables)"
            # "Obtain second set of options and initialize the respective controls/indicators"
            n48 = call "Batch Detect.vi"("Unit ID (A)"=w324, "error in"=w304, "VISA Session In"=w305) -> ("error out"=w334:errorcluster, "Batching available"=w316:bool, "VISA Session Out"=w333:refnum<visa-resource-name>)  [unwired: 6 in]
            n49 = Increment(x=w336) -> (x+1=w319:i32)
            n50 = call "Read Measurement Format.vi"("Unit ID (A)"=w324, "error in"=w334, "VISA Session In"=w333) -> ("error out"=w327:errorcluster, "Data Frame Format"=w329:T27, "VISA Session Out"=w328:refnum<visa-resource-name>)  [unwired: 6 in]
            n51 = Unbundle(w330) -> ("Enabled"=w321:T26, "Disabled and Grayed Out"=w322:T26)
            n52 = Unbundle(w329) -> ("Absolute Pressure"=w301:bool, "Gauge/Diff. Pressure"=w300:bool, "Barometric Pressure"=w299:bool, "Temperature"=w293:bool, "Volumetric"=w294:bool, "Mass"=w295:bool, "Valve Drive"=w292:bool, "Totalizer"=w291:bool, "Totalizer Timer"=w290:bool, "Totalizer Average Flow"=w296:bool, "Totalizer Peak Flow"=w289:bool, "Gas Selected"=w297:bool)  [unwired: 2 out]
            n53 = Or(x=w301, y=w300) -> (x .or. y?=w298:bool)
            n54 = Bundle(cluster=T20 {"Pressure(s)"=TRUE, "Temperature"=TRUE, "Volumetric"=TRUE, "Mass"=TRUE, "Totalizer Average Flow"=FALSE, "Gas Selected"=TRUE} ("Enables: \nData frame and Display"), "Pressure(s)"=w298, "Temperature"=w293, "Volumetric"=w294, "Mass"=w295, "Totalizer Average Flow"=w296, "Gas Selected"=w297) -> (w332:T20)
            n55 = Bundle(cluster=T2 {"Valve Drive"=FALSE, "Totalizer"=TRUE, "Totalizer Timer"=FALSE, "Totalizer Peak Flow"=FALSE, "Show Abs., Gauge\nand Baro. pressures"=FALSE} ("Enables: Data frame only"), "Valve Drive"=w292, "Totalizer"=w291, "Totalizer Timer"=w290, "Totalizer Peak Flow"=w289, "Show Abs., Gauge\nand Baro. pressures"=w299) -> (w288:T2)
            n56 = call "Read Controller Info.vi"("Unit ID (A)"=w324, "error in"=w327, "Software Version"=w307, "VISA Session In"=w328) -> ("error out"=w326:errorcluster, "Disabled Items\n(used with\"DisabledItems[]\" in the\nController Select property node)"=w285:i32[], "Controller Info out"=w306:T14, "VISA Session Out"=w325:refnum<visa-resource-name>)  [unwired: 4 in]
            n57 = Unbundle By Name(w306) -> ("Controller Full Scale"=→"(Full Scale)":dbl, "Controller Select"=w320:u16)
            n58 = property on="Serial and Display" class="Clust (strict)"("Value"=w332) -> ()  [unwired: 2 in, 2 out]
            n59 = property on="Serial Only" class="Clust (strict)"("Value"=w288) -> ()  [unwired: 2 in, 2 out]
            n60 = property on="Controller Select" class="Ring (strict)"("Disabled Items []"=w285) -> ()  [unwired: 2 in, 2 out]
            n61 = Not Equal?(x=w320, y=w287) -> (x != y?=w315:bool)
            n62 = And(x=w316, y=w315) -> (x .and. y?=w314:bool)
            n63 = Select(t=w321, s=w314, f=w322) -> (s? t:f=w335:T26)
            n64 = Select(t=w321, s=w315, f=w322) -> (s? t:f=w323:T26)
            n65 = property on="Batch Setpoint" class="DigNum (strict)"("DisabledEnum"=w335) -> ()  [unwired: 2 in, 2 out]
            n66 = property on="Setpoint" class="DigNum (strict)"("DisabledEnum"=w323) -> ()  [unwired: 2 in, 2 out]
          }
          frame 3 {
            # "Get Totalizer info and check which tare functions are allowable"
            # "Obtain the third set of options and initialize the respective controls/indicators"
            n67 = call "Flow and Pressure Function Check.vi"("Unit ID (A)"=w349, "error in"=w371, "Software Version"=w338, "VISA Session In"=w370) -> ("error out"=w367:errorcluster, "Flow Tare Enabled"=w360:bool, "Pressure Tare Enabled"=w359:bool, "VISA Session Out"=w366:refnum<visa-resource-name>)  [unwired: 4 in]
            n68 = Increment(x=w351) -> (x+1=w350:i32)
            n69 = Unbundle(w363) -> ("Enabled"=w346:T26, "Disabled and Grayed Out"=w345:T26)
            n70 = call "Read Totalizer Units and Decimals.vi"("Unit ID (A)"=w349, "error in"=w367, "Software Version"=w338, "VISA Session In"=w366) -> ("error out"=w354:errorcluster, "Totalizer"=w364:T10, "VISA Session Out"=w353:refnum<visa-resource-name>, "Totalizer decimal places"=w369:i32)  [unwired: 3 in, 1 out]
            "Totalizer" <- w364
            n71 = To Unsigned Byte Integer(number=w369) -> (unsigned 8bit integer=w368:u8)
            n72 = Select(t=w346, s=w359, f=w345) -> (s? t:f=w362:T26)
            n73 = Select(t=w346, s=w360, f=w345) -> (s? t:f=w361:T26)
            n74 = property on="Batch Setpoint" class="DigNum (strict)"("Precision"=w368) -> ()  [unwired: 2 in, 2 out]
            n75 = property on="Tare Pressure" class="Bool"("DisabledEnum"=w362) -> ()  [unwired: 2 in, 2 out]
            n76 = property on="Tare Flow" class="Bool"("DisabledEnum"=w361) -> ()  [unwired: 2 in, 2 out]
            n77 = Not Equal?(x=w364, y=T10."No Totalizer" ("Totalizer")) -> (x != y?=w357:bool)
            n78 = Select(t=w346, s=w357, f=w345) -> (s? t:f=w358:T26)
            n79 = property on="Reset Total" class="Bool"("DisabledEnum"=w358) -> ()  [unwired: 2 in, 2 out]
          }
          frame 4 {
            # "Initialize controller and tare options, and determine if they need to be disabled"
            # "Obtain the fourth set of options and initialize the respective controls/indicators"
            n80 = call "Read Tare Settings.vi"("Unit ID (A)"=w399, "error in"=w391, "VISA Session In"=w390) -> ("error out"=w384:errorcluster, "Tare Functions"=w398:T9, "VISA Session Out"=w385:refnum<visa-resource-name>)  [unwired: 6 in]
            n81 = Increment(x=w411) -> (x+1=w409:i32)
            n82 = Unbundle(w410) -> ("Enabled"=w394:T26, "Disabled and Grayed Out"=w393:T26)
            n83 = Unbundle(w398) -> ("Display"=w395:enum16{"None", "Pressure", "Volumetric"}, "External"=w396:T28, "Auto-Tare Delay [s]"=w397:dbl)
            n84 = Select(t=w394, s=w392, f=w393) -> (s? t:f=w373:T26)
            n85 = property on="Display" class="Enum (strict)"("Value"=w395) -> ()  [unwired: 2 in, 2 out]
            n86 = property on="External" class="Enum (strict)"("Value"=w396) -> ()  [unwired: 2 in, 2 out]
            n87 = property on="Auto-Tare Delay [s]" class="DigNum (strict)"("Value"=w397, "DisabledEnum"=w373) -> ()  [unwired: 2 in, 2 out]
            n88 = call "Read PID Info.vi"("VISA Session In"=w385, "error in"=w384, "Unit ID (A)"=w399) -> ("VISA Session Out"=w388:refnum<visa-resource-name>, "PID Settings"=w405:T29, "error out"=w389:errorcluster)  [unwired: 5 in]
            n89 = Unbundle(w405) -> ("PID Type"=w404:enum8{"PDF", "PD2I"}, "Valve Offset"=w403:i32, "P Gain"=w402:i32, "D Gain"=w401:i32, "I Gain"=w400:i32)  [unwired: 1 out]
            n90 = property on="PID Type" class="Enum (strict)"("Value"=w404, "DisabledEnum"=w373) -> ()  [unwired: 2 in, 2 out]
            n91 = property on="P Gain" class="DigNum (strict)"("Value"=w402, "DisabledEnum"=w373) -> ()  [unwired: 2 in, 2 out]
            n92 = property on="I Gain" class="DigNum (strict)"("Value"=w400, "DisabledEnum"=w373) -> ()  [unwired: 2 in, 2 out]
            n93 = property on="Valve \nOffset" class="DigNum (strict)"("Value"=w403, "DisabledEnum"=w373) -> ()  [unwired: 2 in, 2 out]
            n94 = property on="D Gain" class="DigNum (strict)"("Value"=w401, "DisabledEnum"=w373) -> ()  [unwired: 2 in, 2 out]
            n95 = call "Read Output Definitions and Controller Options.vi"("Unit ID (A)"=w399, "error in"=w389, "Software Version"=w376, "VISA Session In"=w388) -> ("error out"=w387:errorcluster, "Read-Only Options"=→"Read-Only Options":T8, "Read/Write Options"=w377:T1, "VISA Session Out"=w386:refnum<visa-resource-name>)  [unwired: 4 in]
            n96 = Unbundle(w377) -> ("Controller Select"=w372:u16, "SetPoint Source"=w374:enum8{"Serial", "Local", "Analog", "Unknown"}, "AutoTare"=w375:enum16{"Disabled", "Enabled"})
            n97 = property on="Controller Select" class="Ring (strict)"("Value"=w372, "DisabledEnum"=w373) -> ()  [unwired: 2 in, 2 out]
            n98 = property on="SetPoint Source" class="Enum (strict)"("Value"=w374, "DisabledEnum"=w373) -> ()  [unwired: 2 in, 2 out]
            n99 = property on="AutoTare" class="Enum (strict)"("Value"=w375, "DisabledEnum"=w373) -> ()  [unwired: 2 in, 2 out]
          }
          frame 5 {
            w437 = 60.0 ("Pressure")
            # "This VI can not tell if the range is bi-directional or 0 to (-) full scale. This is due to how those are handled in the software.\n As this does not affect the data output, it should not be an issue other than needing to use the auto-scale features of LabVIEW."
            # "Update the chart to have the proper full scales"
            n100 = call "Read Controllable Fullscale Values.vi"("Unit ID (A)"=w424, "error in"=w431, "Software Version"=w430, "VISA Session In"=w432) -> ("error out"=w426:errorcluster, "Fullscale"=w420:T30, "VISA Session Out"=w427:refnum<visa-resource-name>)  [unwired: 5 in]
            n101 = Increment(x=w443) -> (x+1=w442:i32)
            n102 = Unbundle By Name(w441) -> ("Controller Select"=w440:u16)
            n103 = call "Read Register.vi"("Unit ID (A)"=w424, "error in"=w426, "Register address"=u16 38, "VISA Session In"=w427) -> ("error out"=w428:errorcluster, "Register Value (I32)"=w422:i32, "VISA Session Out"=w429:refnum<visa-resource-name>)  [unwired: 5 in]
            n104 = Unbundle(w420) -> ("Absolute Pressure"=w418:dbl, "Gauge/Diff. Pressure"=w417:dbl, "Volumetric Flow"=w415:dbl, "Mass Flow"=w414:dbl)
            n105 = And(x=w422, y=1) -> (x .and. y?=w421:i32)
            n106 = Not Equal To 0?(x=w421) -> (x != 0?=w419:bool)
            n107 = Select(t=w418, s=w419, f=w417) -> (s? t:f=w416:dbl)
            n108 = Build Array(w416, w437, w415, w414, w437) -> (w438:dbl[])
            n109 = Unbundle By Name(w436) -> ("Chart: AutoScale"=w435:bool)
            n110 = for {
              tunnel: w440 -> [w464]
              tunnel: w438 -> [w459] mode=indexing
              tunnel: [w458] -> _
              i -> [w462]
              # "Set each plot's Y scale, sequentially"
              n111 = Equal?(x=4, y=w462) -> (x = y?=w460:bool)
              n112 = To Unsigned Long Integer(number=w462) -> (unsigned 32bit integer=w461:u32)
              n113 = case shown="True" w460 {
                tunnel: w464 -> [_ w471]
                tunnel: w461 -> [w468 w470]
                tunnel: w459 -> [w466 _]
                tunnel: [u32 0 ("Active Plot") w469] -> w458
                frame False {
                  # "Set the Y scale ranges"
                  n114 = property on="Chart" class="WFChart (strict)"("Active Plot"=w468, "YScale.Maximum"=w466, "YScale.Minimum"=0.0 ("Y Scale.Range:Minimum")) -> ()  [unwired: 2 in, 2 out]
                }
                frame True {
                  # "Associate the setpoint scale properly"
                  n115 = case shown="0, Default" w471 {
                    tunnel: [u32 0 ("Active Plot") u32 0 ("Active Plot") u32 1 ("Active Plot") u32 1 ("Active Plot")] -> w469
                    frame 0, Default {
                    }
                    frame 34, 38, 39 {
                      # "Get setpoint scale"
                    }
                    frame 36 {
                    }
                    frame 37 {
                    }
                  }
                  n116 = property on="Chart" class="WFChart (strict)"("Active Plot"=w470, "Plot.YScaleIdx"=w469) -> ()  [unwired: 2 in, 2 out]
                }
              }
            }
            n117 = case shown="True" w435 {
              frame False {
              }
              frame True {
                w452 = u8 2 ("Y Scale.Scale Fit")
                # "AutoScale is true"
                n118 = property on="Chart" class="WFChart (strict)"("Active Plot"=u32 0, "YScale.ScaleFit"=w452, "Active Plot"=u32 1, "YScale.ScaleFit"=w452, "Active Plot"=u32 2, "YScale.ScaleFit"=w452, "Active Plot"=u32 3, "YScale.ScaleFit"=w452, "Active Plot"=u32 4, "YScale.ScaleFit"=w452) -> ()  [unwired: 2 in, 2 out]
              }
            }
          }
          frame 6 {
            w487 = FALSE ("Visible")
            # "Generate Logging info, hide initialization notification, and re-enable updates to the front panel (and close the related references)"
            n119 = property on="Data Logging Options" class="Clust (strict)"() -> ("Value"=w476:T3)  [unwired: 2 in, 2 out]
            n120 = Increment(x=w481) -> (x+1=w482:i32)
            n121 = Unbundle By Name(w476) -> ("Log Data"=w479:bool)
            n122 = case shown="True" w479 {
              tunnel: ["" w509] -> w492
              frame False {
              }
              frame True {
                n123 = Get Date/Time In Seconds() -> (seconds since 1Jan1904=w515:timestamp)
                n124 = Format Date/Time String(time format string (%c)="%m-%d-%Y_%H-%M-%S", seconds (now)=w515) -> (date/time string=w514:string)  [unwired: 1 in]
                n125 = call <vilib>:"Application Directory.vi"() -> ("Application Directory"=w511:path)
                n126 = Format Date/Time String(time format string (%c)="%p", seconds (now)=w515) -> (date/time string=w513:string)  [unwired: 1 in]
                n127 = Path To String(path=w511) -> (string=w508:string)
                n128 = Concatenate Strings(w508, "\\Alicat Data Log_" ("string"), w514, "_" ("string"), w513, ".txt" ("string")) -> (w509:string)
              }
            }
            n129 = call "Data Logging_Generate Header.vi"("error in"=w494, "Include Units\nin Header (F)"=TRUE ("Include Units\nin Header (default is F)"), "Units of Measure Input"=w493, "Data Logging Options"=w476) -> ("error out"=w490:errorcluster, "Data Log Header"=w488:string)  [unwired: 5 in, 1 out]
            n130 = String To Path(string=w492) -> (path=w491:path)
            n131 = case shown="True" w479 {
              tunnel: w491 -> [_ w526]
              tunnel: w490 -> [w519 w525]
              tunnel: [w519 w523] -> w489
              tunnel: w488 -> [_ w522]
              tunnel: [refnum<file> refnum ("refnum out") w521] -> w486
              tunnel: T21."replace or create" ("operation (0:open)") -> [_ w520]
              frame False {
              }
              frame True {
                n132 = Open/Create/Replace File(file path (use dialog)=w526, error in=w525, operation (0:open)=w520) -> (refnum out=w527:refnum<file>, error out=w524:errorcluster)  [unwired: 3 in, 1 out]
                n133 = Write to Text File(file (use dialog)=w527, text=w522, error in=w524) -> (refnum out=w521:refnum<file>, error out=w523:errorcluster)  [unwired: 1 in, 1 out]
              }
            }
            n134 = Unbundle(w499) -> ("Panel"=w497:refnum<vi>)  [unwired: 1 out]
            n135 = property on="Wait message" class="Clust (strict)"(error in=w489, "Visible"=w487) -> (error out=w498:errorcluster)  [unwired: 1 in, 1 out]
            n136 = property class="Pnl"(reference=w497, error in=w498, "DeferPanUpdts"=w487) -> (error out=w483:errorcluster)  [unwired: 1 out]
          }
          frame 7, Default {
            w549 = TRUE ("Data Changed")
            # "No incrementing, this is the data collection state"
            # "Update setpoint control\nto current value on 1st run"
            # "Acquire data"
            # "Data collection"
            n137 = Wait (ms)(milliseconds to wait="Time between \nreadings [ms]") -> ()  [unwired: 1 out]
            n138 = call "Read Measurements.vi"("error in"=w565, "Data Frame Format In"=w564, "Unit ID (A)"=w560, "VISA Session In"=w566) -> ("error out"=w558:errorcluster, "Data Frame Format Out"=w545:T27, "Data Cluster"=w580:T31, "VISA Session Out"=w559:refnum<visa-resource-name>, "Unknown Dataframe Info"=w561:bool, "Error/Overrange/Unknown String"=w529:string, "Error Present"=w562:bool, "Range Exceeded"=w541:bool)
            n139 = Or(x=w561, y=w562) -> (x .or. y?=w540:bool)
            n140 = Unbundle(w580) -> ("Absolute Pressure"=w567:dbl, "Gauge/Diff. Pressure"=w568:dbl, "Barometric Pressure"=w569:dbl, "Temperature"=w570:dbl, "Volumetric Flow"=w554:dbl, "Mass Flow"=w571:dbl, "Setpoint"=w544:dbl, "Valve Drive"=w572:dbl, "Totalizer"=w573:dbl, "[hr]"=w574:dbl, "[min]"=w575:dbl, "[sec]"=w576:dbl, "Totalizer Average Flow"=w577:dbl, "Totalizer Peak Flow"=w543:dbl, "Gas selected"=w542:string)
            n141 = Unbundle(w563) -> ("Abs. Pressure"=w539:string, "Gauge/Diff. Press."=w535:string, "Barometric Press."=w534:string, "Temperature"=w536:string, "Volume"=w533:string, "Mass"=w532:string, "Setpoint"=w530:string, "Valve Drive"=w528:string, "Totalizer"=w531:string, "Tot. Avg. Flow"=w537:string, "Tot. Peak Flow"=w538:string)  [unwired: 1 out]
            n142 = Bundle(cluster=w579, "Absolute Pressure"=w567, "Gauge/Diff. Pressure"=w568, "Barometric Pressure"=w569, "Temperature"=w570, "Volumetric Flow"=w554, "Mass Flow"=w571, "Setpoint"=w544, "Valve Drive"=w572, "Totalizer"=w573, "[h]"=w574, "[m]"=w575, "[s]"=w576, "Totalizer Average Flow"=w577, "Totalizer Peak Flow"=w543, "Gas selected"=w542, "Range Exceeded"=w541, "Error Present"=w540, "ERR/OVR Text"=w529, "Abs. Pressure"=w539, "Temperature 2"=w536, "Volume"=w533, "Mass"=w532, "Totalizer 2"=w531, "Valve Drive 2"=w528, "Gauge/Diff. Press."=w535, "Barometric Press."=w534, "Setpoint 2"=w530, "Tot. Avg. Flow"=w537, "Tot. Peak Flow"=w538) -> (w578:T15)
            n143 = case shown="False" w548 {
              tunnel: w544 -> [w581 _]
              frame False {
                n144 = property on="Setpoint" class="DigNum (strict)"("Value"=w581) -> ()  [unwired: 2 in, 2 out]
              }
              frame True {
              }
            }
          }
        }
        n145 = Select(t=0, s=w171, f=w173) -> (s? t:f=w172:i32)
      }
      event Panel Close? {
        w599 = TRUE ("Discard?")
        # "Discard a panel close command and force the program to end (forces references to be closed before exiting)"
        n146 = event-data() -> ()  [unwired: 1 in, 1 out]
        n147 = event-data("Discard?"=w599) -> ()  [unwired: 1 in, 1 out]
      }
      event "COM Port Settings.VISA Sesssion In": Value Change {
        # "Re-initialize VI"
        # "Close the VISA session and re-initialize it with the new COM port value. Then, it resets the state to 0 to initialize the device"
        n148 = event-data() -> ("NewVal"=w600:refnum<visa-resource-name>)  [unwired: 1 in]
        n149 = VISA Close(VISA resource name=w612, error in (no error)=w613) -> (error out=w614:errorcluster)
        n150 = property on="Baud Rate" class="Enum (strict)"() -> ("Value"=w601:T32)  [unwired: 2 in, 2 out]
        n151 = Bundle(cluster=T12 {"Unit ID"="A", "Baud Rate"=enum."19200", "VISA Sesssion In"="COM1"} ("Communication Settings"), "Unit ID"="A", "Baud Rate"=w601, "VISA Sesssion In"=w600) -> (w603:T12)
        n152 = call "COM Port Initialization.vi"("error in (no error)"=w614, "Communication Settings"=w603) -> ("error out"=w617:errorcluster, "VISA Session Out"=w616:refnum<visa-resource-name>)  [unwired: 8 in]
      }
      event "COM Port Settings.Baud Rate": Value Change {
        # "Re-initialize VI"
        # "Changes the baud rate to match updated value, then it resets the state to 0 to initialize the device"
        n153 = event-data() -> ("NewVal"=w633:T32)  [unwired: 1 in]
        n154 = case shown="\"38400\"" w633 {
          tunnel: [u32 2400 ("Serial Settings:Baud Rate") u32 9600 ("Serial Settings:Baud Rate") u32 19200 ("Serial Settings:Baud Rate") u32 38400 ("Serial Settings:Baud Rate") u32 57600 ("Serial Settings:Baud Rate") u32 11520 ("Serial Settings:Baud Rate") u32 19200 ("Serial Settings:Baud Rate")] -> w632
          frame "2400", Default {
          }
          frame "9600" {
          }
          frame "19200" {
          }
          frame "38400" {
          }
          frame "57600" {
          }
          frame "115200" {
          }
          frame "Unknown" {
          }
        }
        n155 = property class="Serial Instr"(reference=w635, error in=w637, "Baud"=w632) -> (reference out=w634:refnum<visa-resource-name>, error out=w636:errorcluster)
      }
      event "COM Port Settings.Unit ID": Value Change {
        # "Re-initialize VI"
        # "Changes the unit ID to the new value, and then it resets the state to 0 to initialize the device"
        n156 = event-data() -> ("NewVal"=w660:string)  [unwired: 1 in]
      }
      event "Tare Flow": Value Change {
        # "Reset to 0 if\ncomm error\nis present"
        # "Executes the flow tare sub-VI and checks to make sure that the communication to the unit is still established"
        n157 = event-data() -> ()  [unwired: 1 in, 1 out]
        n158 = call "Tare Flow.vi"("Unit ID (A)"=w677, "error in"=w681, "VISA Session In"=w678) -> ("error out"=w680:errorcluster, "VISA Session Out"=w679:refnum<visa-resource-name>)  [unwired: 7 in]
        n159 = Select(t=0, s=w680, f=w682) -> (s? t:f=w683:i32)
      }
      event "Tare Pressure": Value Change {
        # "Reset to 0 if\ncomm error\nis present"
        # "Executes the pressure tare sub-VI and checks to make sure that the communication to the unit is still established"
        n160 = event-data() -> ()  [unwired: 1 in, 1 out]
        n161 = call "Tare Pressure.vi"("Unit ID (A)"=w698, "error in"=w702, "VISA Session In"=w699) -> ("error out"=w701:errorcluster, "VISA Session Out"=w700:refnum<visa-resource-name>)  [unwired: 7 in]
        n162 = Select(t=0, s=w701, f=w703) -> (s? t:f=w704:i32)
      }
      event "Tare AP Sensor": Value Change {
        # "Reset to 0 if\ncomm error\nis present"
        # "Executes the pressure tare sub-VI and checks to make sure that the communication to the unit is still established"
        n163 = event-data() -> ()  [unwired: 1 in, 1 out]
        n164 = call "Tare AP Sensor with Internal Barometer.vi"("Unit ID (A)"=w719, "error in"=w723, "VISA Session In"=w720) -> ("error out"=w722:errorcluster, "VISA Session Out"=w721:refnum<visa-resource-name>)  [unwired: 7 in]
        n165 = Select(t=0, s=w722, f=w724) -> (s? t:f=w725:i32)
      }
      event "Reset Total": Value Change {
        # "Reset to 0 if\ncomm error\nis present"
        # "Executes the Totalizer reset sub-VI and checks to make sure that the communication to the unit is still established"
        n166 = event-data() -> ()  [unwired: 1 in, 1 out]
        n167 = call "Reset Totalizer.vi"("Unit ID (A)"=w740, "error in"=w744, "VISA Session In"=w741) -> ("error out"=w743:errorcluster, "VISA Session Out"=w742:refnum<visa-resource-name>)  [unwired: 6 in, 1 out]
        n168 = Select(t=0, s=w743, f=w745) -> (s? t:f=w746:i32)
      }
      event "Tare Options": Value Change {
        # "Reset to 0 if\ncomm error\nis present"
        # "Writes the new tare settings and checks to make sure that the communication to the unit is still established"
        n169 = event-data() -> ()  [unwired: 1 in, 1 out]
        n170 = call "Write Tare Settings.vi"("Unit ID (A)"=w761, "error in"=w763, "Tare Functions"="Tare Options", "VISA Session In"=w766) -> ("error out"=w764:errorcluster, "VISA Session Out"=w765:refnum<visa-resource-name>)  [unwired: 6 in]
        n171 = Select(t=0, s=w764, f=w767) -> (s? t:f=w768:i32)
      }
      event "Gas Select": Value Change {
        # "Reset to 0 if\ncomm error\nis present"
        # "Writes the new gas selection and checks to make sure that the communication to the unit is still established"
        n172 = event-data() -> ()  [unwired: 1 in, 1 out]
        n173 = call "Write Gas Selection.vi"("Unit ID (A)"=w784, "error in"=w785, "Gas Number"="Gas Select", "VISA Session In"=w788) -> ("error out"=w786:errorcluster, "VISA Session Out"=w787:refnum<visa-resource-name>)  [unwired: 6 in]
        n174 = Select(t=0, s=w786, f=w789) -> (s? t:f=w790:i32)
      }
      event "Read/Write Options": Value Change {
        # "Disallow changing of control variable \nto \"no controller\" if it is a controller.\nAlso, discard invalid choices and notify user"
        # "Reset to 0 if\ncomm error\nis present"
        # "Writes the new controller options (if allowable) and checks to make sure that the communication to the unit is still established"
        n175 = event-data() -> ()  [unwired: 1 in, 6 out]
        n176 = Unbundle By Name(w819) -> ("Controller Select"=w811:u16)
        n177 = Unbundle("Read/Write Options") -> ("Controller Select"=w812:u16, "SetPoint Source"=w818:enum8{"Serial", "Local", "Analog", "Unknown"}, "AutoTare"=w817:enum16{"Disabled", "Enabled"})
        n178 = call "Controller Select_Check Validity.vi"("Software Version"=w800, "Controller?"=w806, "Unit ID (A)"=w805, "error in"=w830, "Controller Select_Old"=w811, "Controller Select_New"=w812, "VISA Session In"=w810) -> ("error out"=w808:errorcluster, "Invalid selection"=w807:bool, "Validated Controller Select"=w798:u16, "VISA Session Out"=w809:refnum<visa-resource-name>)  [unwired: 1 in]
        n179 = Bundle(cluster="Read/Write Options", "Controller Select"=w798, "SetPoint Source"=w818, "AutoTare"=w817) -> (w816:T1)
        n180 = call "Write Controller Options.vi"("Unit ID (A)"=w805, "error in"=w808, "Software Version"=w800, "Read/Write Options"=w816, "VISA Session In"=w809) -> ("error out"=w820:errorcluster, "VISA Session Out"=w821:refnum<visa-resource-name>)  [unwired: 5 in]
        n181 = case shown="0, Default" w798 {
          tunnel: [u32 0 ("Active Plot") u32 0 ("Active Plot") u32 1 ("Active Plot") u32 1 ("Active Plot")] -> w799
          frame 0, Default {
          }
          frame 34, 38, 39 {
            # "Get setpoint scale"
          }
          frame 36 {
          }
          frame 37 {
          }
        }
        n182 = property on="Chart" class="WFChart (strict)"("Active Plot"=u32 4, "Plot.YScaleIdx"=w799) -> ()  [unwired: 2 in, 2 out]
        n183 = call "Display Message to User4"("Enable"=w807) -> ()  [unwired: 9 in, 2 out]
        n184 = Select(t=0, s=w820, f=w822) -> (s? t:f=w823:i32)
      }
      event "PID Settings.P Gain", "PID Settings.D Gain", "PID Settings.I Gain": Value Change {
        # "Reset to 0 if\ncomm error\nis present"
        # "Writes the new PID settings and checks to make sure that the communication to the unit is still established"
        n185 = event-data() -> ()  [unwired: 1 in, 1 out]
        n186 = Unbundle("PID Settings") -> ("P Gain"=w848:i32, "D Gain"=w847:i32, "I Gain"=w846:i32)  [unwired: 2 out]
        n187 = Bundle(cluster=T22 {"P Gain"=0, "D Gain"=0, "I Gain"=0} ("PID Gain Settings"), "P Gain"=w848, "D Gain"=w847, "I Gain"=w846) -> (w850:T22)
        n188 = call "Write PID Gains.vi"("VISA Session In"=w851, "PID Gain Settings"=w850, "error in"=w852, "Unit ID (A)"=w843) -> ("VISA Session Out"=w845:refnum<visa-resource-name>, "error out"=w844:errorcluster)  [unwired: 5 in]
        n189 = Select(t=0, s=w844, f=w853) -> (s? t:f=w854:i32)
      }
      event "PID Settings.PID Type", "PID Settings.Valve \nOffset": Value Change {
        # "Reset to 0 if\ncomm error\nis present"
        # "Writes the new PID settings and checks to make sure that the communication to the unit is still established"
        n190 = event-data() -> ()  [unwired: 1 in, 6 out]
        n191 = property on="PID Settings" class="Clust (strict)"() -> ("Value"=w869:T7)  [unwired: 2 in, 2 out]
        n192 = Unbundle(w869) -> ("PID Type"=w874:enum8{"PDF", "PD2I"}, "Valve \nOffset"=w873:i32)  [unwired: 3 out]
        n193 = Bundle(cluster=T23 {"PID Type"=enum."PDF", "Valve Offset"=0} ("PID Loop Settings"), "PID Type"=w874, "Valve Offset"=w873) -> (w872:T23)
        n194 = call "Write PID Settings.vi"("VISA Session In"=w871, "PID Loop Settings"=w872, "error in"=w870, "Unit ID (A)"=w876) -> ("VISA Session Out"=w878:refnum<visa-resource-name>, "error out"=w877:errorcluster)  [unwired: 5 in]
        n195 = Select(t=0, s=w877, f=w879) -> (s? t:f=w880:i32)
      }
      event "COMPOSER gas mix input.Create COMPOSER Mix": Value Change {
        # "Create COMPOSER mix, then re-populate gas select lists"
        # "Reset to 0 if\ncomm error\nis present"
        # "Writes the desired COMPOSER mix (if possible), and checks to make sure that the communication to the unit is still established"
        n196 = event-data() -> ()  [unwired: 1 in, 6 out]
        n197 = Unbundle("COMPOSER gas mix input") -> ("Mix % 1"=w905:dbl, "Include # 1"=w906:bool, "Mix % 2"=w907:dbl, "Include # 2"=w908:bool, "Mix % 3"=w909:dbl, "Include # 3"=w910:bool, "Mix % 4"=w912:dbl, "Include # 4"=w911:bool, "Mix % 5"=w913:dbl, "Include # 5"=w914:bool, "COMPOSER gas 1"=w919:u16, "COMPOSER gas 2"=w918:u16, "COMPOSER gas 3"=w917:u16, "COMPOSER gas 4"=w916:u16, "COMPOSER gas 5"=w915:u16, "Mix #"=w903:u16, "Mix name"=w902:string)  [unwired: 3 out]
        n198 = Bundle(cluster=T24 {"Gas # 1"=236, "Mix % 1"=0.0, "Include # 1"=FALSE, "Gas # 2"=0, "Mix % 2"=0.0, "Include # 2"=FALSE, "Gas # 3"=0, "Mix % 3"=0.0, "Include # 3"=FALSE, "Gas # 4"=0, "Mix % 4"=0.0, "Include # 4"=FALSE, "Gas # 5"=0, "Mix % 5"=0.0, "Include # 5"=FALSE} ("COMPOSER gas mix input"), "Gas # 1"=w919, "Mix % 1"=w905, "Include # 1"=w906, "Gas # 2"=w918, "Mix % 2"=w907, "Include # 2"=w908, "Gas # 3"=w917, "Mix % 3"=w909, "Include # 3"=w910, "Gas # 4"=w916, "Mix % 4"=w912, "Include # 4"=w911, "Gas # 5"=w915, "Mix % 5"=w913, "Include # 5"=w914) -> (w904:T24)
        n199 = call "Write COMPOSER Gas Mix.vi"("Gas mix name"=w902, "Unit ID (A)"=w892, "error in"=w922, "Gas # to store mix as"=w903, "COMPOSER gas mix input"=w904, "VISA Session In"=w923) -> ("error out"=w894:errorcluster, "Completion text"=w901:string, "VISA Session Out"=w895:refnum<visa-resource-name>)  [unwired: 3 in]
        n200 = property on="Completion\ntext" class="Str"("Value"=w901) -> ()  [unwired: 2 in, 2 out]
        n201 = call "Read Gas List.vi"("Unit ID (A)"=w892, "error in"=w894, "VISA Session In"=w895) -> ("error out"=w888:errorcluster, "Gas Selection: Strings and Values"=w889:cluster{"Gas Name":string, "Gas number":u16}[], "VISA Session Out"=w893:refnum<visa-resource-name>)  [unwired: 5 in, 1 out]
        n202 = property on="Gas Select" class="Ring (strict)"("StringsAndValues[]"=w889) -> ()  [unwired: 2 in, 2 out]
        n203 = property on="COMPOSER gas 1" class="Ring (strict)"("StringsAndValues[]"=w889) -> ()  [unwired: 2 in, 2 out]
        n204 = property on="COMPOSER gas 2" class="Ring (strict)"("StringsAndValues[]"=w889) -> ()  [unwired: 2 in, 2 out]
        n205 = property on="COMPOSER gas 3" class="Ring (strict)"("StringsAndValues[]"=w889) -> ()  [unwired: 2 in, 2 out]
        n206 = property on="COMPOSER gas 4" class="Ring (strict)"("StringsAndValues[]"=w889) -> ()  [unwired: 2 in, 2 out]
        n207 = property on="COMPOSER gas 5" class="Ring (strict)"("StringsAndValues[]"=w889) -> ()  [unwired: 2 in, 2 out]
        n208 = Select(t=0, s=w888, f=w924) -> (s? t:f=w925:i32)
      }
      event "Read Register": Value Change {
        w941 = "%d" ("format string")
        # "Reset to 0 if\ncomm error\nis present"
        # "Reads desired register and displays it. Also checks to make sure that the communication to the unit is still established"
        n209 = event-data() -> ()  [unwired: 1 in, 6 out]
        n210 = Format Into String(format string=w941, initial string="R", "Reg. to read") -> (resulting string=w944:string)  [unwired: 1 in, 1 out]
        n211 = call "Read Register.vi"("Unit ID (A)"=w948, "error in"=w949, "Register address"="Reg. to read", "VISA Session In"=w952) -> ("error out"=w950:errorcluster, "Register Value (I32)"=w946:i32, "VISA Session Out"=w951:refnum<visa-resource-name>)  [unwired: 5 in]
        n212 = Concatenate Strings(w944, " = " ("string")) -> (w942:string)
        n213 = Format Into String(format string=w941, initial string=w942, w946) -> (resulting string=→"Register value":string)  [unwired: 1 in, 1 out]
        n214 = Select(t=0, s=w950, f=w953) -> (s? t:f=w954:i32)
      }
      event "Log Register Values": Value Change {
        # "Reset to 0 if\ncomm error\nis present"
        # "Logs the current register values to a text file in the folder containing this VI. Also checks to make sure that the communication to the unit is still established"
        n215 = event-data() -> ()  [unwired: 1 in, 6 out]
        n216 = call "Log Current Register Values.vi"("Unit ID (A)"=w978, "error in"=w979, "VISA Session In"=w981) -> ("error out"=w968:errorcluster, "VISA Session Out"=w980:refnum<visa-resource-name>)  [unwired: 7 in]
        n217 = Get Date/Time String(want seconds? (F)=TRUE) -> (date string=w974:string, time string=w973:string)  [unwired: 2 in]
        n218 = Concatenate Strings(w974, ", " ("string"), w973) -> (w969:string)
        n219 = Concatenate Strings("Register log saved in VI folder." ("Message"), w969) -> (w971:string)
        n220 = call "Display Message to User"("error in (no error)"=w968, "Message"=w971) -> ("error out"=w967:errorcluster)  [unwired: 8 in, 1 out]
        n221 = Select(t=0, s=w967, f=w982) -> (s? t:f=w983:i32)
      }
      event "Batch Setpoint": Value Change {
        # "Reset to 0 if\ncomm error\nis present"
        # "Writes a new batch setpoint and checks to make sure that the communication to the unit is still established"
        n222 = event-data() -> ()  [unwired: 1 in, 1 out]
        n223 = call "Legacy Detector.vi"("Unit ID (A)"=w991, "error in"=w995, "VISA Session In"=w996) -> ("error out"=w994:errorcluster, "Legacy Status"=w992:u8, "VISA Session Out"=w993:refnum<visa-resource-name>)  [unwired: 6 in]
        n224 = call "Write Batch Setpoint.vi"("Unit ID (A)"=w991, "error in"=w994, "Batch SetPoint"="Batch Setpoint", "Legacy Status"=w992, "VISA Session In"=w993) -> ("error out"=w1004:errorcluster, "VISA Session Out"=w1006:refnum<visa-resource-name>)  [unwired: 5 in]
        n225 = Select(t=0, s=w1004, f=w1007) -> (s? t:f=w1008:i32)
      }
      event "Setpoint": Value Change {
        # "Reset to 0 if\ncomm error\nis present"
        # "Writes new setpoint if different from old setpoint, then parses the returned data frame and checks to make sure that the communication to the unit is still established"
        n226 = event-data() -> ("NewVal"=w1017:dbl)  [unwired: 1 in]
        n227 = call "Write SetPoint.vi"("Setpoint"=w1017, "Previous Setpoint"=w1070, "Unit ID (A)"=w1023, "error in"=w1072, "Software Version"=w1016, "Controller Info out"=w1065, "VISA Session In"=w1073) -> ("error out"=w1068:errorcluster, "Data frame returned"=w1020:string, "Controller Info out"=w1064:T14, "VISA Session Out"=w1025:refnum<visa-resource-name>)  [unwired: 1 in]
        n228 = call "Parse Data Frame.vi"("VISA Session In"=w1025, "Unit ID (A)"=w1023, "Data Frame Input"=w1020, "Data Frame Format In"=w1019, "error in"=w1068, "Offset (2 if polling, 0 if streaming)"=u32 2) -> ("Range Exceeded"=w1027:bool, "Error/Overrange/Unknown String"=w1028:string, "VISA Session Out"=w1024:refnum<visa-resource-name>, "Data Cluster"=w1031:T33, "Data Frame Format Out"=w1018:T13, "Error Present"=w1066:bool, "Unknown Dataframe Info"=w1067:bool, "error out"=w1063:errorcluster)  [unwired: 2 in]
        n229 = Or(x=w1067, y=w1066) -> (x .or. y?=w1026:bool)
        n230 = Unbundle(w1031) -> ("Absolute Pressure"=w1046:dbl, "Gauge/Diff. Pressure"=w1047:dbl, "Barometric Pressure"=w1048:dbl, "Temperature"=w1049:dbl, "Volumetric Flow"=w1045:dbl, "Mass Flow"=w1050:dbl, "Setpoint"=w1044:dbl, "Valve Drive"=w1051:dbl, "Totalizer"=w1052:dbl, "[hr]"=w1053:dbl, "[min]"=w1054:dbl, "[sec]"=w1055:dbl, "Totalizer Average Flow"=w1056:dbl, "Totalizer Peak Flow"=w1043:dbl, "Gas selected"=w1042:string)
        n231 = Unbundle(w1030) -> ("Abs. Pressure"=w1041:string, "Gauge/Diff. Press."=w1037:string, "Barometric Press."=w1036:string, "Temperature"=w1038:string, "Volume"=w1035:string, "Mass"=w1034:string, "Setpoint"=w1032:string, "Valve Drive"=w1029:string, "Totalizer"=w1033:string, "Tot. Avg. Flow"=w1039:string, "Tot. Peak Flow"=w1040:string)  [unwired: 1 out]
        n232 = Bundle(cluster=w1022, "Absolute Pressure"=w1046, "Gauge/Diff. Pressure"=w1047, "Barometric Pressure"=w1048, "Temperature"=w1049, "Volumetric Flow"=w1045, "Mass Flow"=w1050, "Setpoint"=w1044, "Valve Drive"=w1051, "Totalizer"=w1052, "[h]"=w1053, "[m]"=w1054, "[s]"=w1055, "Totalizer Average Flow"=w1056, "Totalizer Peak Flow"=w1043, "Gas selected"=w1042, "Range Exceeded"=w1027, "Error Present"=w1026, "ERR/OVR Text"=w1028, "Abs. Pressure"=w1041, "Temperature 2"=w1038, "Volume"=w1035, "Mass"=w1034, "Totalizer 2"=w1033, "Valve Drive 2"=w1029, "Gauge/Diff. Press."=w1037, "Barometric Press."=w1036, "Setpoint 2"=w1032, "Tot. Avg. Flow"=w1039, "Tot. Peak Flow"=w1040) -> (w1021:T15)
        n233 = property on="Time between \nreadings [ms]" class="DigNum (strict)"() -> ("Value"=w1060:u32)  [unwired: 2 in, 2 out]
        n234 = Wait (ms)(milliseconds to wait=w1060) -> ()  [unwired: 1 out]
        n235 = Select(t=0, s=w1063, f=w1074) -> (s? t:f=w1075:i32)
      }
      event "Serial and Display", "Serial Only": Value Change {
        # "If the requested data frame alteration is not possible, the change will\nbe rejected and the user will be notified."
        # "Reset to 0 if\ncomm error\nis present"
        # "Writes new data frame enables (if allowed), returns the new data frame format cluster, and checks to make sure that the communication to the unit is still established"
        n236 = event-data() -> ()  [unwired: 1 in, 6 out]
        n237 = call "Write Data Frame Options.vi"("Unit ID (A)"=w1113, "error in"=w1119, "Enables: Data frame only"="Serial Only", "Enables: \nData frame and Display"="Serial and Display", "VISA Session In"=w1120) -> ("error out"=w1115:errorcluster, "VISA Session Out"=w1114:refnum<visa-resource-name>)  [unwired: 5 in]
        n238 = call "Read Measurement Format.vi"("Unit ID (A)"=w1113, "error in"=w1115, "VISA Session In"=w1114) -> ("error out"=w1096:errorcluster, "Data Frame Format"=w1111:T27, "VISA Session Out"=w1116:refnum<visa-resource-name>)  [unwired: 6 in]
        n239 = Unbundle(w1111) -> ("Absolute Pressure"=w1091:bool, "Gauge/Diff. Pressure"=w1092:bool, "Barometric Pressure"=w1088:bool, "Temperature"=w1089:bool, "Volumetric"=w1087:bool, "Mass"=w1086:bool, "Valve Drive"=w1083:bool, "Totalizer"=w1082:bool, "Totalizer Timer"=w1081:bool, "Totalizer Average Flow"=w1085:bool, "Totalizer Peak Flow"=w1080:bool, "Gas Selected"=w1084:bool)  [unwired: 2 out]
        n240 = Or(x=w1091, y=w1092) -> (x .or. y?=w1090:bool)
        n241 = Bundle(cluster=T25 {"Pressure"=TRUE, "Temperature"=TRUE, "Volumetric"=TRUE, "Mass"=TRUE, "Totalizer Average Flow"=FALSE, "Gas Selected"=TRUE} ("Serial and Display"), "Pressure"=w1090, "Temperature"=w1089, "Volumetric"=w1087, "Mass"=w1086, "Totalizer Average Flow"=w1085, "Gas Selected"=w1084) -> (w1109:T25)
        n242 = Bundle(cluster=T2 {"Valve Drive"=FALSE, "Totalizer"=TRUE, "Totalizer Timer"=FALSE, "Totalizer Peak Flow"=FALSE, "Show Abs., Gauge\nand Baro. pressures"=FALSE} ("Serial Only"), "Valve Drive"=w1083, "Totalizer"=w1082, "Totalizer Timer"=w1081, "Totalizer Peak Flow"=w1080, "Show Abs., Gauge\nand Baro. pressures"=w1088) -> (w1079:T2)
        n243 = property on="Serial and Display" class="Clust (strict)"("Value"=w1109) -> ()  [unwired: 2 in, 2 out]
        n244 = property on="Serial Only" class="Clust (strict)"("Value"=w1079) -> ()  [unwired: 2 in, 2 out]
        n245 = Not Equal?(x="Serial and Display", y=w1109) -> (x != y?=w1106:T34)
        n246 = Not Equal?(x=w1079, y="Serial Only") -> (x != y?=w1099:T2)
        n247 = Cluster To Array(cluster=w1099) -> (array=w1101:bool[])
        n248 = Cluster To Array(cluster=w1106) -> (array=w1102:bool[])
        n249 = Build Array(w1102, w1101) -> (w1100:bool[][])
        n250 = Boolean To (0,1)(Boolean=w1100) -> (0, 1=w1105:i16[][])
        n251 = Add Array Elements(numeric array=w1105) -> (sum=w1103:i16)
        n252 = Not Equal To 0?(x=w1103) -> (x != 0?=w1104:bool)
        n253 = call "Display Message to User3"("Enable"=w1104) -> ()  [unwired: 9 in, 2 out]
        n254 = Select(t=0, s=w1096, f=w1121) -> (s? t:f=w1122:i32)
      }
      event "Chart: Pressure", "Chart: Temperature", "Chart: Volumetric", "Chart: Mass Flow", "Chart: Graphing", "Chart: Setpoint": Value Change {
        # "Reset to 0 if\ncomm error\nis present"
        # "Adjusts what variables are displayed in the chart, and checks to make sure that the communication to the unit is still established"
        n255 = event-data() -> ()  [unwired: 1 in, 6 out]
        n256 = property on="Chart" class="WFChart (strict)"("Active Plot"=u32 0, "Plot.Visible?"="Chart: Pressure", "Active Plot"=u32 1, "Plot.Visible?"="Chart: Temperature", "Active Plot"=u32 2, "Plot.Visible?"="Chart: Volumetric", "Active Plot"=u32 3, "Plot.Visible?"="Chart: Mass Flow", "Active Plot"=u32 4, "Plot.Visible?"="Chart: Setpoint") -> ()  [unwired: 2 in, 2 out]
        n257 = Select(t=0, s=w1147, f=w1150) -> (s? t:f=w1151:i32)
      }
      event "Chart: AutoScale": Value Change {
        # "Reset to 0 if\ncomm error\nis present"
        # "Toggles the autoscaling depending on the boolean control and checks to make sure that the communication to the unit is still established"
        n258 = event-data() -> ()  [unwired: 1 in, 6 out]
        n259 = case shown="True" "Chart: AutoScale" {
          frame False {
            w1178 = u8 0 ("Y Scale.Scale Fit")
            # "Turn off auto-scaling"
            n260 = property on="Chart" class="WFChart (strict)"("Active Plot"=u32 0, "YScale.ScaleFit"=w1178, "Active Plot"=u32 1, "YScale.ScaleFit"=w1178, "Active Plot"=u32 2, "YScale.ScaleFit"=w1178, "Active Plot"=u32 3, "YScale.ScaleFit"=w1178, "Active Plot"=u32 4, "YScale.ScaleFit"=w1178) -> ()  [unwired: 2 in, 2 out]
          }
          frame True {
            w1184 = u8 2 ("Y Scale.Scale Fit")
            # "AutoScale is true"
            n261 = property on="Chart" class="WFChart (strict)"("Active Plot"=u32 0, "YScale.ScaleFit"=w1184, "Active Plot"=u32 1, "YScale.ScaleFit"=w1184, "Active Plot"=u32 2, "YScale.ScaleFit"=w1184, "Active Plot"=u32 3, "YScale.ScaleFit"=w1184, "Active Plot"=u32 4, "YScale.ScaleFit"=w1184) -> ()  [unwired: 2 in, 2 out]
          }
        }
        n262 = Select(t=0, s=w1167, f=w1170) -> (s? t:f=w1171:i32)
      }
      event "Chart: Manual Scale Adjust": Value Change {
        w1206 = u8 0 ("Y Scale.Scale Fit")
        # "Disable auto-scaling, then go through a menu to set the new scales"
        # "Reset to 0 if\ncomm error\nis present"
        # "Toggles the autoscaling depending on the boolean control and checks to make sure that the communication to the unit is still established"
        n263 = event-data() -> ()  [unwired: 1 in, 1 out]
        n264 = property on="Chart" class="WFChart (strict)"(error in=w1205, "Active Plot"=u32 0, "YScale.ScaleFit"=w1206, "Active Plot"=u32 1, "YScale.ScaleFit"=w1206, "Active Plot"=u32 2, "YScale.ScaleFit"=w1206, "Active Plot"=u32 3, "YScale.ScaleFit"=w1206, "Active Plot"=u32 4, "YScale.ScaleFit"=w1206) -> (error out=w1197:errorcluster)  [unwired: 1 in, 1 out]
        n265 = call <vilib>:"Three Button Dialog.vi"("Allow user to close window? (TRUE)"=FALSE, "Window Title (\"\")"="Scale Adjustment Options" ("Window Title (\"\")"), "Right Button Text (\"Cancel\")"="Cancel" ("Left Button Text (\"Yes\")"), "Center Button Text (\"No\")"="Fit scales to current data" ("Left Button Text (\"Yes\")"), "Left Button Text (\"Yes\")"="Adjust scales manually" ("Left Button Text (\"Yes\")"), "message"="Adjust scales manually, or fit scales to current data?") -> ("Which Button?"=w1198:T35)  [unwired: 5 in]
        n266 = case shown="\"Left Button\", Default" w1198 {
          tunnel: w1197 -> [w1227 w1237 w1244]
          tunnel: [w1227 w1236 w1244] -> w1195
          tunnel: w1191 -> [w1226 _ _]
          frame "Left Button", Default {
            # "Adjust scales manually"
            n267 = call "Scale Adjustment Menu.vi"("Data Frame Format"=w1226) -> ("Scale Minimum"=w1229:dbl, "Scale Maximum"=w1230:dbl, "Active Y scale"=w1231:u32, "Request Cancelled"=w1228:bool)  [unwired: 6 in, 1 out]
            n268 = case shown="False" w1228 {
              tunnel: w1231 -> [w1232 _]
              tunnel: w1230 -> [w1235 _]
              tunnel: w1229 -> [w1234 _]
              frame False {
                # "Adjust scales if false"
                n269 = To Long Integer(number=w1232) -> (32bit integer=w1233:i32)
                n270 = property on="Chart" class="WFChart (strict)"("ActYScl"=w1233, "YScale.Maximum"=w1235, "YScale.Minimum"=w1234) -> ()  [unwired: 2 in, 2 out]
              }
              frame True {
                # "request was aborted"
              }
            }
          }
          frame "Center Button" {
            w1238 = u8 1 ("Y Scale.Scale Fit")
            # "Fit scales to current data"
            n271 = property on="Chart" class="WFChart (strict)"(error in=w1237, "Active Plot"=u32 0, "YScale.ScaleFit"=w1238, "Active Plot"=u32 1, "YScale.ScaleFit"=w1238, "Active Plot"=u32 2, "YScale.ScaleFit"=w1238, "Active Plot"=u32 3, "YScale.ScaleFit"=w1238, "Active Plot"=u32 4, "YScale.ScaleFit"=w1238) -> (error out=w1236:errorcluster)  [unwired: 1 in, 1 out]
          }
          frame "Right Button" {
            # "Request was aborted"
          }
        }
        n272 = property on="Chart: AutoScale" class="Bool (strict)"(error in=w1195, "Value"=FALSE ("Chart: AutoScale")) -> (error out=w1196:errorcluster)  [unwired: 1 in, 1 out]
        n273 = Select(t=0, s=w1196, f=w1218) -> (s? t:f=w1219:i32)
      }
      event "Data Logging Options": Value Change {
        # "Close current data file"
        # "Update the Logging options control with the valid options\n(essentially: throw out bad selections and notify the user)"
        # "Checks validity of choices and disables them if invalid. This also ensures that future data logging calls are using valid data"
        # "Reset to 0 if\ncomm error\nis present"
        # "Closes previously opened file (if applicable), opens a new one, and checks to make sure that the communication to the unit is still established"
        n274 = event-data() -> ()  [unwired: 1 in, 1 out]
        n275 = case shown="True" w1249 {
          tunnel: w1252 -> [_ w1281]
          tunnel: w1251 -> [w1278 w1280]
          tunnel: [w1278 w1279] -> w1250
          frame False {
          }
          frame True {
            n276 = Close File(refnum=w1281, error in=w1280) -> (error out=w1279:errorcluster)  [unwired: 1 out]
          }
        }
        n277 = Unbundle By Name("Data Logging Options") -> ("Log Data"=w1253:bool)
        n278 = case shown="True" w1253 {
          tunnel: ["" w1295] -> w1266
          frame False {
          }
          frame True {
            n279 = Get Date/Time In Seconds() -> (seconds since 1Jan1904=w1301:timestamp)
            n280 = Format Date/Time String(time format string (%c)="%m-%d-%Y_%H-%M-%S", seconds (now)=w1301) -> (date/time string=w1300:string)  [unwired: 1 in]
            n281 = call <vilib>:"Application Directory.vi"() -> ("Application Directory"=w1297:path)
            n282 = Format Date/Time String(time format string (%c)="%p", seconds (now)=w1301) -> (date/time string=w1299:string)  [unwired: 1 in]
            n283 = Path To String(path=w1297) -> (string=w1294:string)
            n284 = Concatenate Strings(w1294, "\\Alicat Data Log_" ("string"), w1300, "_" ("string"), w1299, ".txt" ("string")) -> (w1295:string)
          }
        }
        n285 = call "Data Logging_Check Validity.vi"("error in"=w1250, "Data Frame Format"=w1256, "Data Logging Options (If valid)"="Data Logging Options") -> ("error out"=w1258:errorcluster, "Invalid data selected"=w1257:bool, "Validated Logging Options"=w1245:T3)  [unwired: 6 in]
        n286 = property on="Data Logging Options" class="Clust (strict)"("Value"=w1245) -> ()  [unwired: 2 in, 2 out]
        n287 = call "Data Logging_Generate Header.vi"("error in"=w1258, "Include Units\nin Header (F)"=TRUE ("Include Units\nin Header (default is F)"), "Units of Measure Input"=w1259, "Data Logging Options"=w1245) -> ("error out"=w1264:errorcluster, "Data Log Header"=w1263:string)  [unwired: 5 in, 1 out]
        n288 = String To Path(string=w1266) -> (path=w1262:path)
        n289 = case shown="True" w1253 {
          tunnel: [w1283 w1289] -> w1265
          tunnel: w1264 -> [w1283 w1284]
          tunnel: w1263 -> [_ w1288]
          tunnel: w1262 -> [_ w1287]
          tunnel: T21."replace or create" ("operation (0:open)") -> [_ w1286]
          tunnel: [refnum<file> refnum ("refnum out") w1285] -> w1260
          frame False {
          }
          frame True {
            n290 = Open/Create/Replace File(file path (use dialog)=w1287, error in=w1284, operation (0:open)=w1286) -> (refnum out=w1291:refnum<file>, error out=w1290:errorcluster)  [unwired: 3 in, 1 out]
            n291 = Write to Text File(file (use dialog)=w1291, text=w1288, error in=w1290) -> (refnum out=w1285:refnum<file>, error out=w1289:errorcluster)  [unwired: 1 in, 1 out]
          }
        }
        n292 = call "Display Message to User2"("Enable"=w1257) -> ()  [unwired: 9 in, 2 out]
        n293 = Select(t=0, s=w1265, f=w1271) -> (s? t:f=w1272:i32)
      }
    }
    n294 = case shown="True" w70 {
      selector: w70 -> [w99 _]
      tunnel: w73 -> [_ w112]
      tunnel: [w99 FALSE ("Data Changed")] -> w71
      tunnel: w69 -> [w97 w113]
      tunnel: w68 -> [w98 w124]
      tunnel: [w98 w123] -> w67
      tunnel: [w97 w103] -> w51
      tunnel: w65 -> [w96 w120]
      tunnel: [w96 w119] -> w66
      tunnel: w55 -> [_ w114]
      tunnel: w47 -> [_ w102]
      frame False {
      }
      frame True {
        # "Only update if new data is received, only log or plot if enabled"
        n295 = case shown="True" w114 {
          tunnel: w124 -> [w129 w154]
          tunnel: [w129 w153] -> w123
          tunnel: w113 -> [w128 w152]
          tunnel: w112 -> [w127 w147]
          tunnel: [w128 w148] -> w103
          tunnel: [w127 w147] -> w111
          frame False {
          }
          frame True {
            # "If true: generate data\nstring and log it to file"
            n296 = local read "Data Logging Options"() -> (w150:T3)
            n297 = Unbundle(w147) -> ("Absolute Pressure"=w146:dbl, "Gauge/Diff. Pressure"=w145:dbl, "Barometric Pressure"=w144:dbl, "Temperature"=w143:dbl, "Volumetric Flow"=w142:dbl, "Mass Flow"=w141:dbl, "Setpoint"=w140:dbl, "Valve Drive"=w139:dbl, "Totalizer"=w138:dbl, "[h]"=w137:dbl, "[m]"=w136:dbl, "[s]"=w135:dbl, "Totalizer Average Flow"=w131:dbl, "Totalizer Peak Flow"=w132:dbl, "Gas selected"=w133:string)  [unwired: 14 out]
            n298 = Bundle(cluster=T19 {"Absolute Pressure"=0.0, "Gauge/Diff. Pressure"=0.0, "Barometric Pressure"=0.0, "Temperature"=0.0, "Volumetric"=0.0, "Mass Flow"=0.0, "Setpoint"=0.0, "Valve Drive"=0.0, "Totalizer"=0.0, "[hr]"=0.0, "[min]"=0.0, "[sec]"=0.0, "Totalizer Average Flow"=0.0, "Totalizer Peak Flow"=0.0, "Gas selected"=""} ("Measurement Data"), "Absolute Pressure"=w146, "Gauge/Diff. Pressure"=w145, "Barometric Pressure"=w144, "Temperature"=w143, "Volumetric"=w142, "Mass Flow"=w141, "Setpoint"=w140, "Valve Drive"=w139, "Totalizer"=w138, "[hr]"=w137, "[min]"=w136, "[sec]"=w135, "Totalizer Average Flow"=w131, "Totalizer Peak Flow"=w132, "Gas selected"=w133) -> (w130:T19)
            n299 = call "Data Logging_Generate Data String.vi"("error in"=w152, "Measurement Data"=w130, "Data Logging Options"=w150) -> ("error out"=w149:errorcluster, "Data Log String"=w151:string)  [unwired: 6 in, 1 out]
            n300 = Write to Text File(file (use dialog)=w154, text=w151, error in=w149) -> (refnum out=w153:refnum<file>, error out=w148:errorcluster)  [unwired: 1 in, 1 out]
          }
        }
        "Measurement Data" <- w111
        n301 = Unbundle By Name(w102) -> ("Absolute Pressure"=w101:bool)
        n302 = Unbundle By Name(w111) -> ("Absolute Pressure"=w109:dbl, "Gauge/Diff. Pressure"=w100:dbl, "Temperature"=w107:dbl, "Volumetric Flow"=w106:dbl, "Mass Flow"=w105:dbl, "Setpoint"=w104:dbl)
        n303 = call "Elapsed Time"("Set Start Time (s)"=w120) -> ("Get Start Time (s)"=w119:dbl, "Elapsed Time (s)"=w116:dbl)  [unwired: 11 in, 6 out]
        n304 = Select(t=w109, s=w101, f=w100) -> (s? t:f=w108:dbl)
        n305 = Multiply(x=1000.0, y=w116) -> (x*y=→"Time between\nreadings [ms]":dbl)
        n306 = Reciprocal(x=w116) -> (1/x=→"Meas. per\nsecond [Hz]":dbl)
        n307 = Bundle(cluster=T5 {"Pressure"=0.0, "Temperature"=0.0, "Volumetric"=0.0, "Mass"=0.0, "SetPoint"=0.0} ("Chart"), "Pressure"=w108, "Temperature"=w107, "Volumetric"=w106, "Mass"=w105, "SetPoint"=w104) -> (w122:T5)
        n308 = case shown="True" "Chart: Graphing" {
          tunnel: w122 -> [_ w126]
          frame False {
          }
          frame True {
            "Chart" <- w126
          }
        }
      }
    }
    n309 = Select(t=50, s=w51, f=0) -> (s? t:f=w59:i32)
    n310 = Select(t=w51, s=w51, f=w49) -> (s? t:f=w50:errorcluster)
  }
  n311 = case shown="True" w7 {
    tunnel: w26 -> [_ w1304]
    frame False {
    }
    frame True {
      # "Currently logging"
      n312 = Close File(refnum=w1304) -> ()  [unwired: 1 in, 2 out]
    }
  }
  n313 = Unbundle(w12) -> (w11:refnum<vi>, "Panel"=w10:refnum<vi>)
  n314 = VISA Close(VISA resource name=w45, error in (no error)=w43) -> (error out=w14:errorcluster)
  n315 = Close Reference(reference=w11, error in (no error)=w14) -> (error out=w15:errorcluster)
  n316 = Close Reference(reference=w10, error in (no error)=w15) -> (error out=w13:errorcluster)
  n317 = call <vilib>:"Simple Error Handler.vi"("error in (no error)"=w13) -> ()  [unwired: 4 in, 5 out]
